vi "Database Viewer.vi"() -> ()   [LabVIEW 2019, in "Database Viewer.lvclass"]
doc: "- key stroke \"Left\" = \"Ctrl\" + \"Left\", \"Right\" = \"Ctrl\" + \"Right\" since left and right arror key are often used and using them for event will intertere with cursor movement.\n- drag cursor will update the start and end\n- load favorite A by Ctrl + A (?)\n- load favorite B by Ctrl + B (?)\n- load favorite C by Ctrl + C (?)"
uses:
  Database Viewer.lvclass
  typedefs/Time Mode--enum.ctl
  typedefs/Time Bucket--enum.ctl
  <vilib>/Utility/miscctls.llb/LVRangeTypeDef.ctl
  <userlib>/LevyLab/Instrument Framework/SMOs/Configuration/Configuration.lvclass
  typedefs/UI Controls--cluster.ctl
  Database Viewer.lvclass/Database Viewer.ctl
  <vilib>/Utility/miscctls.llb/LVRectTypeDef.ctl
  <vilib>/Utility/sysdir.llb/System Directory Type.ctl
  <userlib>/_OpenG.lib/array/array.llb/Index 1D Array Elements (String)__ogtk.vi
  <userlib>/LevyLab/LV-Data/LV-Data.PG/LV-Data.PGSQL.lvclass
  <userlib>/LevyLab/LV-Data/LV-Data.ITX/LV-Data.ITX.lvclass
  <userlib>/LevyLab/Instrument Framework/SMOs/Instrument/Instrument.lvclass
panel:
  in  "Disconnect":bool
  in  "Exit":bool
  out "Status":string
  in  "Time Bucket":T1=enum."automatic"
  out "Get Trace SQL":string
  in  "Execute Custom SQL?":bool
  in  "SQL String":string
  in  "Y Scale Mapping (Right)":enum16{"linear", "log"}(ring)
  in  "Max Points":i32=1000
  in  "Y Scale Mapping (Left)":enum16{"linear", "log"}(ring)
  in  "Median Filter?":bool
  in  "Favorite":enum16{"A", "B", "C"}(ring)
  in  "DST":bool=TRUE caption="Blank Button"
  in  "Variables (left axis)":u16[](array[ring]) caption="Display the following network shared variables (Left / Y)" items=["ALEX_DEMO: DEMO (discoveries)", "AML Gauges (Analysis): Emission Current (A)", "AML Gauges (Analysis): Fault ()", "AML Gauges (Analysis): IG Pressure (mbar)", "AML Gauges (Analysis): Instrument Status ()", "AML Gauges (Analysis): Pirani 1 Pressure (mbar)", "AML Gauges (Analysis): Pirani 2 Pressure (mbar)", "AML Gauges (Analysis): Relay A ()", "AML Gauges (Analysis): Relay B ()", "AML Gauges (Analysis): Relay C ()", "AML Gauges (Analysis): Relay D ()", "AML Gauges (Analysis): Trip A Association ()", "AML Gauges (Analysis): Trip A Pressure (mbar)", "AML Gauges (Analysis): Trip B Association ()", "AML Gauges (Analysis): Trip B Pressure (mbar)", "AML Gauges (Analysis): Trip C Association ()", "AML Gauges (Analysis): Trip C Pressure (mbar)", "AML Gauges (Analysis): Trip D Association ()", "AML Gauges (Analysis): Trip D Pressure (mbar)", "AML Gauges (Prep): Emission Current (A)", "AML Gauges (Prep): Fault ()", "AML Gauges (Prep): IG Pressure (mbar)", "AML Gauges (Prep): Instrument Status ()", "AML Gauges (Prep): Pirani 1 Pressure (mbar)", "AML Gauges (Prep): Pirani 2 Pressure (mbar)", "AML Gauges (Prep): Relay A ()", "AML Gauges (Prep): Relay B ()", "AML Gauges (Prep): Relay C ()", "AML Gauges (Prep): Relay D ()", "AML Gauges (Prep): Trip A Association ()", "AML Gauges (Prep): Trip A Pressure (mbar)", "AML Gauges (Prep): Trip B Association ()", "AML Gauges (Prep): Trip B Pressure (mbar)", "AML Gauges (Prep): Trip C Association ()", "AML Gauges (Prep): Trip C Pressure (mbar)", "AML Gauges (Prep): Trip D Association ()", "AML Gauges (Prep): Trip D Pressure (mbar)", "ASEQSpectra: Spectra ()", "Agilent AFM: Device ()", "Agilent AFM: Tip Voltage (volts)", "Agilent AFM: User ()", "Agilent AFM: X Pos (a.u.)", "Agilent AFM: Y Pos (a.u.)", "Agilent AFM: Z Pos (a.u.)", "CL SMS 18: Field (T)", "CL SMS 18: He Level (mm)", "CL SMS 18: Rate ()", "CL SMS 18: Target (T)", "CL SMS 18: Voltage (V)", "Colby: Delay (ps)", "Cypher: Comments ()", "Cypher: Device ()", "Cypher: Status ()", "Cypher: User ()", "DR200: 100 mK Plate R (Ohm)", "DR200: 100 mK Plate T (K)", "DR200: 4K Head R X55749 (Ohm)", "DR200: 4K Head R X55750 (Ohm)", "DR200: 4K Head T X55749 (K)", "DR200: 4K Head T X55750 (K)", "DR200: 70K Head R PT100 1 (Ohm)", "DR200: 70K Head R PT100 2 (Ohm)", "DR200: 70K Head T PT100 1 (K)", "DR200: 70K Head T PT100 2 (K)", "DR200: Dewar Pressure (mbar)", "DR200: Forepump Pressure (mbar)", "DR200: MC Heater (W)", "DR200: MC R RuO2 (Ohm)", "DR200: MC R X55751 (Ohm)", "DR200: MC T RuO2 (K)", "DR200: MC T X55751 (K)", "DR200: Mag Bottom R X48230 (Ohm)", "DR200: Mag Bottom R X52698 (Ohm)", "DR200: Mag Bottom T X48230 (K)", "DR200: Mag Bottom T X52698 (K)", "DR200: Mag Top R X48230 (Ohm)", "DR200: Mag Top R X52698 (Ohm)", "DR200: Mag Top T X48230 (K)", "DR200: Mag Top T X52698 (K)", "DR200: Magnet Field (T)", "DR200: Magnet Field Target (T)", "DR200: Magnet PS Current (A)", "DR200: Magnet PS Field (T)", "DR200: Magnet PS Voltage (V)", "DR200: Magnet Status Activity ()", "DR200: Magnet Status Mode ()", "DR200: Magnet Status Switch Heater ()", "DR200: Magnet Status System ()", "DR200: Magnet Target Rate (-)", "DR200: PT Current (A)", "DR200: PT Helium T (C)", "DR200: PT Oil T (C)", "DR200: PT Water In T (C)", "DR200: PT Water Out T (C)", "DR200: PressureFPSafety (Bar)", "DR200: PressureM1Condense (Bar)", "DR200: PressureM3Tank (Bar)", "DR200: Still Heater (W)", "DR200: Still Pressure (mBar)", "DR200: Still R (Ohm)", "DR200: Still T (K)", "Element 2: Diode Current Actual (A)", "Element 2: Diode Current Set (A)", "Element 2: Laser Status ()", "Element 2: Pump Power (W)", "Element 2: Startup/Shutdown Status ()", "Element 2: Temp: Control Unit (C)", "Element 2: Temp: Laser Head Pos1 (C)", "Element 2: Temp: Laser Head Pos2 (C)", "Element 2: Temp: Pump Chassis (C)", "Element 2: Temp: Pump Diodes (C)", "Element 2: Temp: Pump PCB (C)", "Element 2: Temp: Pump Tower (C)", "Gemini2: Device ()", "Gemini2: User ()", "JEOL: Device ()", "JEOL: User ()", "Leiden CF FP: Flow ()", "Leiden CF FP: MaxiGauge1 (mbar)", "Leiden CF FP: MaxiGauge2 (mbar)", "Leiden CF FP: MaxiGauge3 (mbar)", "Leiden CF FP: MaxiGauge4 (mbar)", "Leiden CF FP: MaxiGauge5 (mbar)", "Leiden CF FP: MaxiGauge6 (mbar)", "Leiden CF FP: P1 (mbar)", "Leiden CF FP: P2 (mbar)", "Leiden CF FP: P3 (mbar)", "Leiden CF FP: P4 (mbar)", "Leiden CF FP: P5 (mbar)", "Leiden CF FP: P6 (mbar)", "Leiden CF FP: P7 (mbar)", "Leiden CF FP: PT Current (A)", "Leiden CF FP: PT Helium T (C)", "Leiden CF FP: PT Oil T (C)", "Leiden CF FP: PT On ()", "Leiden CF FP: PT P High (bar)", "Leiden CF FP: PT P Low (bar)", "Leiden CF FP: PT Water In T (C)", "Leiden CF FP: PT Water Out T (C)", "Leiden CF FP: STATE ()", "Leiden CF FP: state0 ()", "Leiden CF FP: state1 ()", "Leiden CF FP: state2 ()", "Leiden CF900: CF FP P1 (no_idea)", "Leiden CF900: CF_TC_I0 (Amp)", "Leiden CF900: CF_TC_I1 (Amp)", "Leiden CF900: CF_TC_I2 (Amp)", "Leiden CF900: CF_TC_I3 (Amp)", "Leiden CF900: CF_TC_R0 (ohms)", "Leiden CF900: CF_TC_R1 (ohms)", "Leiden CF900: CF_TC_R2 (ohms)", "Leiden CF900: CF_TC_R3 (ohms)", "Leiden CF900: CF_TC_R4 (ohms)", "Leiden CF900: CF_TC_R5 (ohms)", "Leiden CF900: CF_TC_R6 (ohms)", "Leiden CF900: CF_TC_R7 (ohms)", "Leiden CF900: CF_TC_T0 (mK)", "Leiden CF900: CF_TC_T1 (mK)", "Leiden CF900: CF_TC_T2 (mK)", "Leiden CF900: CF_TC_T3 (mK)", "Leiden CF900: CF_TC_T4 (mK)", "Leiden CF900: CF_TC_T5 (mK)", "Leiden CF900: CF_TC_T6 (mK)", "Leiden CF900: CF_TC_T7 (mK)", "Leiden CF900: CF_TC_Z_R0 (ohms)", "Leiden CF900: CF_TC_Z_R1 (ohms)", "Leiden CF900: CF_TC_Z_R2 (ohms)", "Leiden CF900: CF_TC_Z_R3 (ohms)", "Leiden CF900: CF_TC_Z_R4 (ohms)", "Leiden CF900: CF_TC_Z_R5 (ohms)", "Leiden CF900: CF_TC_Z_R6 (ohms)", "Leiden CF900: CF_TC_Z_R7 (ohms)", "Leiden CF900: CF_TC_Z_R8 (ohms)", "Leiden CF900: CF_TC_Z_R9 (ohms)", "Leiden CF900: CF_TC_Z_T0 (mK)", "Leiden CF900: CF_TC_Z_T1 (mK)", "Leiden CF900: CF_TC_Z_T2 (mK)", "Leiden CF900: CF_TC_Z_T3 (mK)", "Leiden CF900: CF_TC_Z_T4 (mK)", "Leiden CF900: CF_TC_Z_T5 (mK)", "Leiden CF900: CF_TC_Z_T6 (mK)", "Leiden CF900: CF_TC_Z_T7 (mK)", "Leiden CF900: CF_TC_Z_T8 (mK)", "Leiden CF900: CF_TC_Z_T9 (mK)", "Leiden CF900: CF_TC_Z_calibration ()", "Leiden CF900: CF_TC_Z_description ()", "Leiden CF900: CF_TC_calibration ()", "Leiden CF900: CF_TC_description ()", "Leiden CF900: Device ()", "Leiden CF900: User ()", "Leiden MNK Front Panel: Flow ()", "Leiden MNK Front Panel: MaxiGauge1 (mbar)", "Leiden MNK Front Panel: MaxiGauge2 (mbar)", "Leiden MNK Front Panel: MaxiGauge3 (mbar)", "Leiden MNK Front Panel: MaxiGauge4 (mbar)", "Leiden MNK Front Panel: MaxiGauge5 (mbar)", "Leiden MNK Front Panel: MaxiGauge6 (mbar)", "Leiden MNK Front Panel: P1 (mbar)", "Leiden MNK Front Panel: P2 (mbar)", "Leiden MNK Front Panel: P3 (mbar)", "Leiden MNK Front Panel: P4 (mbar)", "Leiden MNK Front Panel: P5 (mbar)", "Leiden MNK Front Panel: P6 (mbar)", "Leiden MNK Front Panel: P7 (mbar)", "Leiden MNK Front Panel: STATE ()", "Leiden MNK Front Panel: state0 ()", "Leiden MNK Front Panel: state1 ()", "Leiden MNK Front Panel: state2 ()", "MFP3D: Device ()", "MFP3D: User ()", "MNK_18T: Device ()", "MNK_18T: IPS Command ()", "MNK_18T: IPS Current (A)", "MNK_18T: IPS IPS Voltage (V)", "MNK_18T: IPS LHe (%)", "MNK_18T: IPS LN2 (%)", "MNK_18T: IPS M1 Current (A)", "MNK_18T: IPS M1 Voltage (V)", "MNK_18T: IPS M2 Current (A)", "MNK_18T: IPS M2 Voltage (V)", "MNK_18T: IPS M3 Current (A)", "MNK_18T: IPS M3 Voltage (V)", "MNK_18T: IPS Magnet Field (T)", "MNK_18T: IPS PS Field (T)", "MNK_18T: IPS Reply ()", "MNK_18T: IPS Status ()", "MNK_18T: IPS Switch ()", "MNK_18T: IPS Target Field (T)", "MNK_18T: IPS Target Field Rate (T/min)", "MNK_18T: IPS Temperature (K)", "MNK_18T: IPS Temperature Resistance (Ohms)", "MNK_18T: ITC Command ()", "MNK_18T: ITC Needle Valve (%)", "MNK_18T: ITC Pressure (mbar)", "MNK_18T: ITC Reply ()", "MNK_18T: ITC Temperature (K)", "MNK_18T: ITC Temperature R (Ohms)", "MNK_18T: MNK_CMN-187_T (mK)", "MNK_18T: MNK_CMN-187_Z (H)", "MNK_18T: MNK_Cstill_T (mK)", "MNK_18T: MNK_Cstill_Z (pF)", "MNK_18T: MNK_TC_I0 (Amp)", "MNK_18T: MNK_TC_I1 (Amp)", "MNK_18T: MNK_TC_I2 (Amp)", "MNK_18T: MNK_TC_I3 (Amp)", "MNK_18T: MNK_TC_R0 (ohms)", "MNK_18T: MNK_TC_R1 (ohms)", "MNK_18T: MNK_TC_R2 (ohms)", "MNK_18T: MNK_TC_R3 (ohms)", "MNK_18T: MNK_TC_R4 (ohms)", "MNK_18T: MNK_TC_R5 (ohms)", "MNK_18T: MNK_TC_R6 (ohms)", "MNK_18T: MNK_TC_R7 (ohms)", "MNK_18T: MNK_TC_T0 (mK)", "MNK_18T: MNK_TC_T1 (mK)", "MNK_18T: MNK_TC_T2 (mK)", "MNK_18T: MNK_TC_T3 (mK)", "MNK_18T: MNK_TC_T4 (mK)", "MNK_18T: MNK_TC_T5 (mK)", "MNK_18T: MNK_TC_T6 (mK)", "MNK_18T: MNK_TC_T7 (mK)", "MNK_18T: MNK_TC_calibration ()", "MNK_18T: MNK_TC_description ()", "MNK_18T: User ()", "Montana Cryostation: Alarm State ()", "Montana Cryostation: Case Valve State ()", "Montana Cryostation: Chamber Pressure (mTorr)", "Montana Cryostation: Cold Head Speed (Hz)", "Montana Cryostation: Compressor Return Pressure (MPa)", "Montana Cryostation: Compressor Run State ()", "Montana Cryostation: Compressor Speed (Hz)", "Montana Cryostation: Compressor Supply Pressure (MPa)", "Montana Cryostation: Device ()", "Montana Cryostation: Idle State ()", "Montana Cryostation: Nitrogen State ()", "Montana Cryostation: Platform Heater Power (W)", "Montana Cryostation: Platform Stability (K)", "Montana Cryostation: Platform Temperature (K)", "Montana Cryostation: Sample Stability (K)", "Montana Cryostation: Sample Temperature (K)", "Montana Cryostation: Stage 1 Heater Power (W)", "Montana Cryostation: Stage 1 Temperature (K)", "Montana Cryostation: Stage 2 Heater Power (W)", "Montana Cryostation: Stage 2 Temperature (K)", "Montana Cryostation: Temperature Set Point (K)", "Montana Cryostation: User ()", "Montana Cryostation: User Stability (K)", "Montana Cryostation: User Temperature (K)", "Montana Cryostation: User Temperature Set Point (K)", "Montana Cryostation: Vent Valve State ()", "Oxford VRM: Current PSU 1 (A)", "Oxford VRM: Current PSU 2 (A)", "Oxford VRM: Current PSU 3 (A)", "Oxford VRM: Current PSU 4 (A)", "Oxford VRM: Current PSU 5 (A)", "Oxford VRM: Current PSU 6 (A)", "Oxford VRM: Current X (A)", "Oxford VRM: Current Y (A)", "Oxford VRM: Current Z (A)", "Oxford VRM: Field X (T)", "Oxford VRM: Field Y (T)", "Oxford VRM: Field Z (T)", "Oxford VRM: IPS Reply ()", "Oxford VRM: Status X ()", "Oxford VRM: Status Y ()", "Oxford VRM: Status Z ()", "Oxford VRM: Target Field Rate X (T/min)", "Oxford VRM: Target Field Rate Y (T/min)", "Oxford VRM: Target Field Rate Z (T/min)", "Oxford VRM: Target Field X (T)", "Oxford VRM: Target Field Y (T)", "Oxford VRM: Target Field Z (T)", "Oxford VRM: Voltage PSU 1 (V)", "Oxford VRM: Voltage PSU 2 (V)", "Oxford VRM: Voltage PSU 3 (V)", "Oxford VRM: Voltage PSU 4 (V)", "Oxford VRM: Voltage PSU 5 (V)", "Oxford VRM: Voltage PSU 6 (V)", "Oxford VRM: Voltage X (V)", "Oxford VRM: Voltage Y (V)", "Oxford VRM: Voltage Z (V)", "PPMS 1: Chamber Status ()", "PPMS 1: Device ()", "PPMS 1: Helium Level (%)", "PPMS 1: Magnet Status ()", "PPMS 1: Magnetic Field (Oe)", "PPMS 1: Position (deg)", "PPMS 1: Temperature (K)", "PPMS 1: Temperature Status ()", "PPMS 1: User ()", "PPMS 2: Chamber Status ()", "PPMS 2: Device ()", "PPMS 2: Helium Level (%)", "PPMS 2: Magnet Status ()", "PPMS 2: Magnetic Field (Oe)", "PPMS 2: Position (deg)", "PPMS 2: Temperature (K)", "PPMS 2: Temperature Status ()", "PPMS 2: User ()", "PPMS 3: Chamber Status ()", "PPMS 3: Device ()", "PPMS 3: Helium Level (%)", "PPMS 3: Magnet Status ()", "PPMS 3: Magnetic Field (T)", "PPMS 3: Temperature (K)", "PPMS 3: Temperature Status ()", "PPMS 3: User ()", "PPMSim: Chamber Status ()", "PPMSim: Device ()", "PPMSim: Helium Level (%)", "PPMSim: Loaded? ()", "PPMSim: Magnet Status ()", "PPMSim: Magnetic Field (T)", "PPMSim: No. of leads (leads)", "PPMSim: Temperature (K)", "PPMSim: Temperature Status ()", "PPMSim: User ()", "PPMSim: v1 (volts)", "PPMSim: v2 (volts)", "PPMSim: v3 (volts)", "Pfeiffer ASM340: Leak Rate (mbar.l/s)", "Pfeiffer ASM340: Pressure (mbar)", "Razorbill: Bridge Capacitance (pF)", "Razorbill: Bridge Excitation (V)", "Razorbill: Bridge Loss (nS)", "Razorbill: Current Ch 1 (A)", "Razorbill: Current Ch 2 (A)", "Razorbill: Level Ch 1 (V)", "Razorbill: Level Ch 2 (V)", "Razorbill: Output State Ch 1 ()", "Razorbill: Output State Ch 2 ()", "Razorbill: Slew Ch 1 (V/s)", "Razorbill: Slew Ch 2 (V/s)", "Razorbill: Voltage Ch 1 (V)", "Razorbill: Voltage Ch 2 (V)", "T/H Monitoring:  (K)", "T/H Monitoring: Astartes_H (%RH)", "T/H Monitoring: Astartes_T (K)", "T/H Monitoring: Centaur_H (%RH)", "T/H Monitoring: Centaur_T (K)", "T/H Monitoring: CustardPie_H (%RH)", "T/H Monitoring: CustardPie_T (K)", "T/H Monitoring: DOT_H (%RH)", "T/H Monitoring: DOT_T (K)", "T/H Monitoring: Griffin_H (%RH)", "T/H Monitoring: Griffin_T (K)", "T/H Monitoring: Kholek_H (%RH)", "T/H Monitoring: Kholek_T (K)", "T/H Monitoring: MFP3D2_H (%RH)", "T/H Monitoring: MFP3D2_T (K)", "T/H Monitoring: MFP3D_H (%RH)", "T/H Monitoring: MFP3D_T (K)", "TEST_TABLE:  (K)", "TEST_TABLE: Columntest2 ()", "TEST_TABLE: Columntest3 ()", "TEST_TABLE: Columntest4 ()", "TEST_TABLE: Custard_T (K)", "TEST_TABLE: Kholek_T (K)", "TEST_TABLE: MFP3D2.phyast.pitt.edu_H (%RH)", "TEST_TABLE: MFP3D2.phyast.pitt.edu_T (K)", "TEST_TABLE: MFP3D2_H (%RH)", "TEST_TABLE: MFP3D2_T (K)", "TEST_TABLE: ON? ()", "TEST_TABLE: Ranjani_H (%)", "TEST_TABLE: Ranjani_T (K)", "TEST_TABLE: Ranjani_new (K)", "TEST_TABLE: Temperature (Kelvin)", "TEST_TABLE: Temperhum_H (%RH)", "TEST_TABLE: Temperhum_T (K)", "TEST_TABLE: Test (tests)", "TEST_TABLE: Test2 (tests)", "TEST_TABLE: _H (%RH)", "TEST_TABLE: _T (K)", "TEST_TABLE: col5 ()", "TEST_TABLE: column2 ()", "TEST_TABLE: connected ()", "TEST_TABLE: ranjani_1 (discoveries)", "TEST_TABLE: sample ()", "TEST_TABLE: test (K)", "TEST_TABLE: testcolumn3 ()", "TEST_TABLE: user ()", "TEST_TABLE: voltaga__demo (volts)", "TEST_TABLE: voltage 2 (volts)", "TEST_TABLE_2: Columntest7 ()", "TEST_TABLE_2: columntest4 ()", "TEST_TABLE_2: new column name (elias)", "TEST_TABLE_2: successfulness (discoveries)", "THz1 SPC: DummyData ()", "Tsunami: Device ()", "Tsunami: User ()"]
  in  "Variables (right axis)":u16[](array[ring]) caption="Display the following network shared variables (Right / X)" items=["ALEX_DEMO: DEMO (discoveries)", "AML Gauges (Analysis): Emission Current (A)", "AML Gauges (Analysis): Fault ()", "AML Gauges (Analysis): IG Pressure (mbar)", "AML Gauges (Analysis): Instrument Status ()", "AML Gauges (Analysis): Pirani 1 Pressure (mbar)", "AML Gauges (Analysis): Pirani 2 Pressure (mbar)", "AML Gauges (Analysis): Relay A ()", "AML Gauges (Analysis): Relay B ()", "AML Gauges (Analysis): Relay C ()", "AML Gauges (Analysis): Relay D ()", "AML Gauges (Analysis): Trip A Association ()", "AML Gauges (Analysis): Trip A Pressure (mbar)", "AML Gauges (Analysis): Trip B Association ()", "AML Gauges (Analysis): Trip B Pressure (mbar)", "AML Gauges (Analysis): Trip C Association ()", "AML Gauges (Analysis): Trip C Pressure (mbar)", "AML Gauges (Analysis): Trip D Association ()", "AML Gauges (Analysis): Trip D Pressure (mbar)", "AML Gauges (Prep): Emission Current (A)", "AML Gauges (Prep): Fault ()", "AML Gauges (Prep): IG Pressure (mbar)", "AML Gauges (Prep): Instrument Status ()", "AML Gauges (Prep): Pirani 1 Pressure (mbar)", "AML Gauges (Prep): Pirani 2 Pressure (mbar)", "AML Gauges (Prep): Relay A ()", "AML Gauges (Prep): Relay B ()", "AML Gauges (Prep): Relay C ()", "AML Gauges (Prep): Relay D ()", "AML Gauges (Prep): Trip A Association ()", "AML Gauges (Prep): Trip A Pressure (mbar)", "AML Gauges (Prep): Trip B Association ()", "AML Gauges (Prep): Trip B Pressure (mbar)", "AML Gauges (Prep): Trip C Association ()", "AML Gauges (Prep): Trip C Pressure (mbar)", "AML Gauges (Prep): Trip D Association ()", "AML Gauges (Prep): Trip D Pressure (mbar)", "ASEQSpectra: Spectra ()", "Agilent AFM: Device ()", "Agilent AFM: Tip Voltage (volts)", "Agilent AFM: User ()", "Agilent AFM: X Pos (a.u.)", "Agilent AFM: Y Pos (a.u.)", "Agilent AFM: Z Pos (a.u.)", "CL SMS 18: Field (T)", "CL SMS 18: He Level (mm)", "CL SMS 18: Rate ()", "CL SMS 18: Target (T)", "CL SMS 18: Voltage (V)", "Colby: Delay (ps)", "Cypher: Comments ()", "Cypher: Device ()", "Cypher: Status ()", "Cypher: User ()", "DR200: 100 mK Plate R (Ohm)", "DR200: 100 mK Plate T (K)", "DR200: 4K Head R X55749 (Ohm)", "DR200: 4K Head R X55750 (Ohm)", "DR200: 4K Head T X55749 (K)", "DR200: 4K Head T X55750 (K)", "DR200: 70K Head R PT100 1 (Ohm)", "DR200: 70K Head R PT100 2 (Ohm)", "DR200: 70K Head T PT100 1 (K)", "DR200: 70K Head T PT100 2 (K)", "DR200: Dewar Pressure (mbar)", "DR200: Forepump Pressure (mbar)", "DR200: MC Heater (W)", "DR200: MC R RuO2 (Ohm)", "DR200: MC R X55751 (Ohm)", "DR200: MC T RuO2 (K)", "DR200: MC T X55751 (K)", "DR200: Mag Bottom R X48230 (Ohm)", "DR200: Mag Bottom R X52698 (Ohm)", "DR200: Mag Bottom T X48230 (K)", "DR200: Mag Bottom T X52698 (K)", "DR200: Mag Top R X48230 (Ohm)", "DR200: Mag Top R X52698 (Ohm)", "DR200: Mag Top T X48230 (K)", "DR200: Mag Top T X52698 (K)", "DR200: Magnet Field (T)", "DR200: Magnet Field Target (T)", "DR200: Magnet PS Current (A)", "DR200: Magnet PS Field (T)", "DR200: Magnet PS Voltage (V)", "DR200: Magnet Status Activity ()", "DR200: Magnet Status Mode ()", "DR200: Magnet Status Switch Heater ()", "DR200: Magnet Status System ()", "DR200: Magnet Target Rate (-)", "DR200: PT Current (A)", "DR200: PT Helium T (C)", "DR200: PT Oil T (C)", "DR200: PT Water In T (C)", "DR200: PT Water Out T (C)", "DR200: PressureFPSafety (Bar)", "DR200: PressureM1Condense (Bar)", "DR200: PressureM3Tank (Bar)", "DR200: Still Heater (W)", "DR200: Still Pressure (mBar)", "DR200: Still R (Ohm)", "DR200: Still T (K)", "Element 2: Diode Current Actual (A)", "Element 2: Diode Current Set (A)", "Element 2: Laser Status ()", "Element 2: Pump Power (W)", "Element 2: Startup/Shutdown Status ()", "Element 2: Temp: Control Unit (C)", "Element 2: Temp: Laser Head Pos1 (C)", "Element 2: Temp: Laser Head Pos2 (C)", "Element 2: Temp: Pump Chassis (C)", "Element 2: Temp: Pump Diodes (C)", "Element 2: Temp: Pump PCB (C)", "Element 2: Temp: Pump Tower (C)", "Gemini2: Device ()", "Gemini2: User ()", "JEOL: Device ()", "JEOL: User ()", "Leiden CF FP: Flow ()", "Leiden CF FP: MaxiGauge1 (mbar)", "Leiden CF FP: MaxiGauge2 (mbar)", "Leiden CF FP: MaxiGauge3 (mbar)", "Leiden CF FP: MaxiGauge4 (mbar)", "Leiden CF FP: MaxiGauge5 (mbar)", "Leiden CF FP: MaxiGauge6 (mbar)", "Leiden CF FP: P1 (mbar)", "Leiden CF FP: P2 (mbar)", "Leiden CF FP: P3 (mbar)", "Leiden CF FP: P4 (mbar)", "Leiden CF FP: P5 (mbar)", "Leiden CF FP: P6 (mbar)", "Leiden CF FP: P7 (mbar)", "Leiden CF FP: PT Current (A)", "Leiden CF FP: PT Helium T (C)", "Leiden CF FP: PT Oil T (C)", "Leiden CF FP: PT On ()", "Leiden CF FP: PT P High (bar)", "Leiden CF FP: PT P Low (bar)", "Leiden CF FP: PT Water In T (C)", "Leiden CF FP: PT Water Out T (C)", "Leiden CF FP: STATE ()", "Leiden CF FP: state0 ()", "Leiden CF FP: state1 ()", "Leiden CF FP: state2 ()", "Leiden CF900: CF FP P1 (no_idea)", "Leiden CF900: CF_TC_I0 (Amp)", "Leiden CF900: CF_TC_I1 (Amp)", "Leiden CF900: CF_TC_I2 (Amp)", "Leiden CF900: CF_TC_I3 (Amp)", "Leiden CF900: CF_TC_R0 (ohms)", "Leiden CF900: CF_TC_R1 (ohms)", "Leiden CF900: CF_TC_R2 (ohms)", "Leiden CF900: CF_TC_R3 (ohms)", "Leiden CF900: CF_TC_R4 (ohms)", "Leiden CF900: CF_TC_R5 (ohms)", "Leiden CF900: CF_TC_R6 (ohms)", "Leiden CF900: CF_TC_R7 (ohms)", "Leiden CF900: CF_TC_T0 (mK)", "Leiden CF900: CF_TC_T1 (mK)", "Leiden CF900: CF_TC_T2 (mK)", "Leiden CF900: CF_TC_T3 (mK)", "Leiden CF900: CF_TC_T4 (mK)", "Leiden CF900: CF_TC_T5 (mK)", "Leiden CF900: CF_TC_T6 (mK)", "Leiden CF900: CF_TC_T7 (mK)", "Leiden CF900: CF_TC_Z_R0 (ohms)", "Leiden CF900: CF_TC_Z_R1 (ohms)", "Leiden CF900: CF_TC_Z_R2 (ohms)", "Leiden CF900: CF_TC_Z_R3 (ohms)", "Leiden CF900: CF_TC_Z_R4 (ohms)", "Leiden CF900: CF_TC_Z_R5 (ohms)", "Leiden CF900: CF_TC_Z_R6 (ohms)", "Leiden CF900: CF_TC_Z_R7 (ohms)", "Leiden CF900: CF_TC_Z_R8 (ohms)", "Leiden CF900: CF_TC_Z_R9 (ohms)", "Leiden CF900: CF_TC_Z_T0 (mK)", "Leiden CF900: CF_TC_Z_T1 (mK)", "Leiden CF900: CF_TC_Z_T2 (mK)", "Leiden CF900: CF_TC_Z_T3 (mK)", "Leiden CF900: CF_TC_Z_T4 (mK)", "Leiden CF900: CF_TC_Z_T5 (mK)", "Leiden CF900: CF_TC_Z_T6 (mK)", "Leiden CF900: CF_TC_Z_T7 (mK)", "Leiden CF900: CF_TC_Z_T8 (mK)", "Leiden CF900: CF_TC_Z_T9 (mK)", "Leiden CF900: CF_TC_Z_calibration ()", "Leiden CF900: CF_TC_Z_description ()", "Leiden CF900: CF_TC_calibration ()", "Leiden CF900: CF_TC_description ()", "Leiden CF900: Device ()", "Leiden CF900: User ()", "Leiden MNK Front Panel: Flow ()", "Leiden MNK Front Panel: MaxiGauge1 (mbar)", "Leiden MNK Front Panel: MaxiGauge2 (mbar)", "Leiden MNK Front Panel: MaxiGauge3 (mbar)", "Leiden MNK Front Panel: MaxiGauge4 (mbar)", "Leiden MNK Front Panel: MaxiGauge5 (mbar)", "Leiden MNK Front Panel: MaxiGauge6 (mbar)", "Leiden MNK Front Panel: P1 (mbar)", "Leiden MNK Front Panel: P2 (mbar)", "Leiden MNK Front Panel: P3 (mbar)", "Leiden MNK Front Panel: P4 (mbar)", "Leiden MNK Front Panel: P5 (mbar)", "Leiden MNK Front Panel: P6 (mbar)", "Leiden MNK Front Panel: P7 (mbar)", "Leiden MNK Front Panel: STATE ()", "Leiden MNK Front Panel: state0 ()", "Leiden MNK Front Panel: state1 ()", "Leiden MNK Front Panel: state2 ()", "MFP3D: Device ()", "MFP3D: User ()", "MNK_18T: Device ()", "MNK_18T: IPS Command ()", "MNK_18T: IPS Current (A)", "MNK_18T: IPS IPS Voltage (V)", "MNK_18T: IPS LHe (%)", "MNK_18T: IPS LN2 (%)", "MNK_18T: IPS M1 Current (A)", "MNK_18T: IPS M1 Voltage (V)", "MNK_18T: IPS M2 Current (A)", "MNK_18T: IPS M2 Voltage (V)", "MNK_18T: IPS M3 Current (A)", "MNK_18T: IPS M3 Voltage (V)", "MNK_18T: IPS Magnet Field (T)", "MNK_18T: IPS PS Field (T)", "MNK_18T: IPS Reply ()", "MNK_18T: IPS Status ()", "MNK_18T: IPS Switch ()", "MNK_18T: IPS Target Field (T)", "MNK_18T: IPS Target Field Rate (T/min)", "MNK_18T: IPS Temperature (K)", "MNK_18T: IPS Temperature Resistance (Ohms)", "MNK_18T: ITC Command ()", "MNK_18T: ITC Needle Valve (%)", "MNK_18T: ITC Pressure (mbar)", "MNK_18T: ITC Reply ()", "MNK_18T: ITC Temperature (K)", "MNK_18T: ITC Temperature R (Ohms)", "MNK_18T: MNK_CMN-187_T (mK)", "MNK_18T: MNK_CMN-187_Z (H)", "MNK_18T: MNK_Cstill_T (mK)", "MNK_18T: MNK_Cstill_Z (pF)", "MNK_18T: MNK_TC_I0 (Amp)", "MNK_18T: MNK_TC_I1 (Amp)", "MNK_18T: MNK_TC_I2 (Amp)", "MNK_18T: MNK_TC_I3 (Amp)", "MNK_18T: MNK_TC_R0 (ohms)", "MNK_18T: MNK_TC_R1 (ohms)", "MNK_18T: MNK_TC_R2 (ohms)", "MNK_18T: MNK_TC_R3 (ohms)", "MNK_18T: MNK_TC_R4 (ohms)", "MNK_18T: MNK_TC_R5 (ohms)", "MNK_18T: MNK_TC_R6 (ohms)", "MNK_18T: MNK_TC_R7 (ohms)", "MNK_18T: MNK_TC_T0 (mK)", "MNK_18T: MNK_TC_T1 (mK)", "MNK_18T: MNK_TC_T2 (mK)", "MNK_18T: MNK_TC_T3 (mK)", "MNK_18T: MNK_TC_T4 (mK)", "MNK_18T: MNK_TC_T5 (mK)", "MNK_18T: MNK_TC_T6 (mK)", "MNK_18T: MNK_TC_T7 (mK)", "MNK_18T: MNK_TC_calibration ()", "MNK_18T: MNK_TC_description ()", "MNK_18T: User ()", "Montana Cryostation: Alarm State ()", "Montana Cryostation: Case Valve State ()", "Montana Cryostation: Chamber Pressure (mTorr)", "Montana Cryostation: Cold Head Speed (Hz)", "Montana Cryostation: Compressor Return Pressure (MPa)", "Montana Cryostation: Compressor Run State ()", "Montana Cryostation: Compressor Speed (Hz)", "Montana Cryostation: Compressor Supply Pressure (MPa)", "Montana Cryostation: Device ()", "Montana Cryostation: Idle State ()", "Montana Cryostation: Nitrogen State ()", "Montana Cryostation: Platform Heater Power (W)", "Montana Cryostation: Platform Stability (K)", "Montana Cryostation: Platform Temperature (K)", "Montana Cryostation: Sample Stability (K)", "Montana Cryostation: Sample Temperature (K)", "Montana Cryostation: Stage 1 Heater Power (W)", "Montana Cryostation: Stage 1 Temperature (K)", "Montana Cryostation: Stage 2 Heater Power (W)", "Montana Cryostation: Stage 2 Temperature (K)", "Montana Cryostation: Temperature Set Point (K)", "Montana Cryostation: User ()", "Montana Cryostation: User Stability (K)", "Montana Cryostation: User Temperature (K)", "Montana Cryostation: User Temperature Set Point (K)", "Montana Cryostation: Vent Valve State ()", "Oxford VRM: Current PSU 1 (A)", "Oxford VRM: Current PSU 2 (A)", "Oxford VRM: Current PSU 3 (A)", "Oxford VRM: Current PSU 4 (A)", "Oxford VRM: Current PSU 5 (A)", "Oxford VRM: Current PSU 6 (A)", "Oxford VRM: Current X (A)", "Oxford VRM: Current Y (A)", "Oxford VRM: Current Z (A)", "Oxford VRM: Field X (T)", "Oxford VRM: Field Y (T)", "Oxford VRM: Field Z (T)", "Oxford VRM: IPS Reply ()", "Oxford VRM: Status X ()", "Oxford VRM: Status Y ()", "Oxford VRM: Status Z ()", "Oxford VRM: Target Field Rate X (T/min)", "Oxford VRM: Target Field Rate Y (T/min)", "Oxford VRM: Target Field Rate Z (T/min)", "Oxford VRM: Target Field X (T)", "Oxford VRM: Target Field Y (T)", "Oxford VRM: Target Field Z (T)", "Oxford VRM: Voltage PSU 1 (V)", "Oxford VRM: Voltage PSU 2 (V)", "Oxford VRM: Voltage PSU 3 (V)", "Oxford VRM: Voltage PSU 4 (V)", "Oxford VRM: Voltage PSU 5 (V)", "Oxford VRM: Voltage PSU 6 (V)", "Oxford VRM: Voltage X (V)", "Oxford VRM: Voltage Y (V)", "Oxford VRM: Voltage Z (V)", "PPMS 1: Chamber Status ()", "PPMS 1: Device ()", "PPMS 1: Helium Level (%)", "PPMS 1: Magnet Status ()", "PPMS 1: Magnetic Field (Oe)", "PPMS 1: Position (deg)", "PPMS 1: Temperature (K)", "PPMS 1: Temperature Status ()", "PPMS 1: User ()", "PPMS 2: Chamber Status ()", "PPMS 2: Device ()", "PPMS 2: Helium Level (%)", "PPMS 2: Magnet Status ()", "PPMS 2: Magnetic Field (Oe)", "PPMS 2: Position (deg)", "PPMS 2: Temperature (K)", "PPMS 2: Temperature Status ()", "PPMS 2: User ()", "PPMS 3: Chamber Status ()", "PPMS 3: Device ()", "PPMS 3: Helium Level (%)", "PPMS 3: Magnet Status ()", "PPMS 3: Magnetic Field (T)", "PPMS 3: Temperature (K)", "PPMS 3: Temperature Status ()", "PPMS 3: User ()", "PPMSim: Chamber Status ()", "PPMSim: Device ()", "PPMSim: Helium Level (%)", "PPMSim: Loaded? ()", "PPMSim: Magnet Status ()", "PPMSim: Magnetic Field (T)", "PPMSim: No. of leads (leads)", "PPMSim: Temperature (K)", "PPMSim: Temperature Status ()", "PPMSim: User ()", "PPMSim: v1 (volts)", "PPMSim: v2 (volts)", "PPMSim: v3 (volts)", "Pfeiffer ASM340: Leak Rate (mbar.l/s)", "Pfeiffer ASM340: Pressure (mbar)", "Razorbill: Bridge Capacitance (pF)", "Razorbill: Bridge Excitation (V)", "Razorbill: Bridge Loss (nS)", "Razorbill: Current Ch 1 (A)", "Razorbill: Current Ch 2 (A)", "Razorbill: Level Ch 1 (V)", "Razorbill: Level Ch 2 (V)", "Razorbill: Output State Ch 1 ()", "Razorbill: Output State Ch 2 ()", "Razorbill: Slew Ch 1 (V/s)", "Razorbill: Slew Ch 2 (V/s)", "Razorbill: Voltage Ch 1 (V)", "Razorbill: Voltage Ch 2 (V)", "T/H Monitoring:  (K)", "T/H Monitoring: Astartes_H (%RH)", "T/H Monitoring: Astartes_T (K)", "T/H Monitoring: Centaur_H (%RH)", "T/H Monitoring: Centaur_T (K)", "T/H Monitoring: CustardPie_H (%RH)", "T/H Monitoring: CustardPie_T (K)", "T/H Monitoring: DOT_H (%RH)", "T/H Monitoring: DOT_T (K)", "T/H Monitoring: Griffin_H (%RH)", "T/H Monitoring: Griffin_T (K)", "T/H Monitoring: Kholek_H (%RH)", "T/H Monitoring: Kholek_T (K)", "T/H Monitoring: MFP3D2_H (%RH)", "T/H Monitoring: MFP3D2_T (K)", "T/H Monitoring: MFP3D_H (%RH)", "T/H Monitoring: MFP3D_T (K)", "TEST_TABLE:  (K)", "TEST_TABLE: Columntest2 ()", "TEST_TABLE: Columntest3 ()", "TEST_TABLE: Columntest4 ()", "TEST_TABLE: Custard_T (K)", "TEST_TABLE: Kholek_T (K)", "TEST_TABLE: MFP3D2.phyast.pitt.edu_H (%RH)", "TEST_TABLE: MFP3D2.phyast.pitt.edu_T (K)", "TEST_TABLE: MFP3D2_H (%RH)", "TEST_TABLE: MFP3D2_T (K)", "TEST_TABLE: ON? ()", "TEST_TABLE: Ranjani_H (%)", "TEST_TABLE: Ranjani_T (K)", "TEST_TABLE: Ranjani_new (K)", "TEST_TABLE: Temperature (Kelvin)", "TEST_TABLE: Temperhum_H (%RH)", "TEST_TABLE: Temperhum_T (K)", "TEST_TABLE: Test (tests)", "TEST_TABLE: Test2 (tests)", "TEST_TABLE: _H (%RH)", "TEST_TABLE: _T (K)", "TEST_TABLE: col5 ()", "TEST_TABLE: column2 ()", "TEST_TABLE: connected ()", "TEST_TABLE: ranjani_1 (discoveries)", "TEST_TABLE: sample ()", "TEST_TABLE: test (K)", "TEST_TABLE: testcolumn3 ()", "TEST_TABLE: user ()", "TEST_TABLE: voltaga__demo (volts)", "TEST_TABLE: voltage 2 (volts)", "TEST_TABLE_2: Columntest7 ()", "TEST_TABLE_2: columntest4 ()", "TEST_TABLE_2: new column name (elias)", "TEST_TABLE_2: successfulness (discoveries)", "THz1 SPC: DummyData ()", "Tsunami: Device ()", "Tsunami: User ()"]
  in  "Export Button":bool
  in  "export path":path=path "C:/Users/Voodoo/Desktop/export"
  out "Shift Hours":dbl=-4.0 format="%#_13g"
  in  "Igor":bool=TRUE caption="Blank Button"
  in  "Connect":bool
  in  "Save Configuration":bool
  in  "Load Configuration":bool
  in  "Mode":T2
  in  "Span":dbl format="%<%D d %H hr %M min %S s>t"
  in  "Trees Visible? >>>>>>":bool
  in  "Tab Control":T3(tab)
  out "Database Time Graph":T4(graph) caption="Retrieved from Citadel 5"
  out "XY Graph":cluster{"data":dbl[], "data":dbl[]}[](graph)
  out "SQL Result":string[][](table)
  out "Trigger Timer (ms)":u32
  out "\"\"":string="Exit\nData: Cleanup\nPostgres: Close Connection\nMacro: Exit\n\nUI: Hide/show trees\nData: Set timeout\nUI: Front Panel State\nUI: Initialize\nInitialize Core Data\nData: Initialize\nMacro: Initialize\r\n"
  in  "Start":dbl format="%<%x %.3X>T"
  in  "End":dbl format="%<%x %.3X>T"
  in  "Seek Back Button":bool
  in  "Seek Forward Button":bool
  in  "Seek":dbl=3600.0 format="%<%H:%M:%S>t"
  in  "Tab Control 2":enum32{"TimeScale - Tree"}(tab)
  in  "postgreSQL Tree (Right / X)":string[](tree)
  in  "postgreSQL Tree (Left / Y)":string[](tree)
  # "Database Connect"
  # "Traces"
  # "Configuration"
  # "Export"
  # "Information: LevyLab Database Viewer v2023.02.17"
  # "Time Axis"
  # "Vertical Axis"
  # "Custom SQL"
  # "Y1\nY2\n.\n.\n."
  # "X1\nX2\n.\n.\n."
  # "."
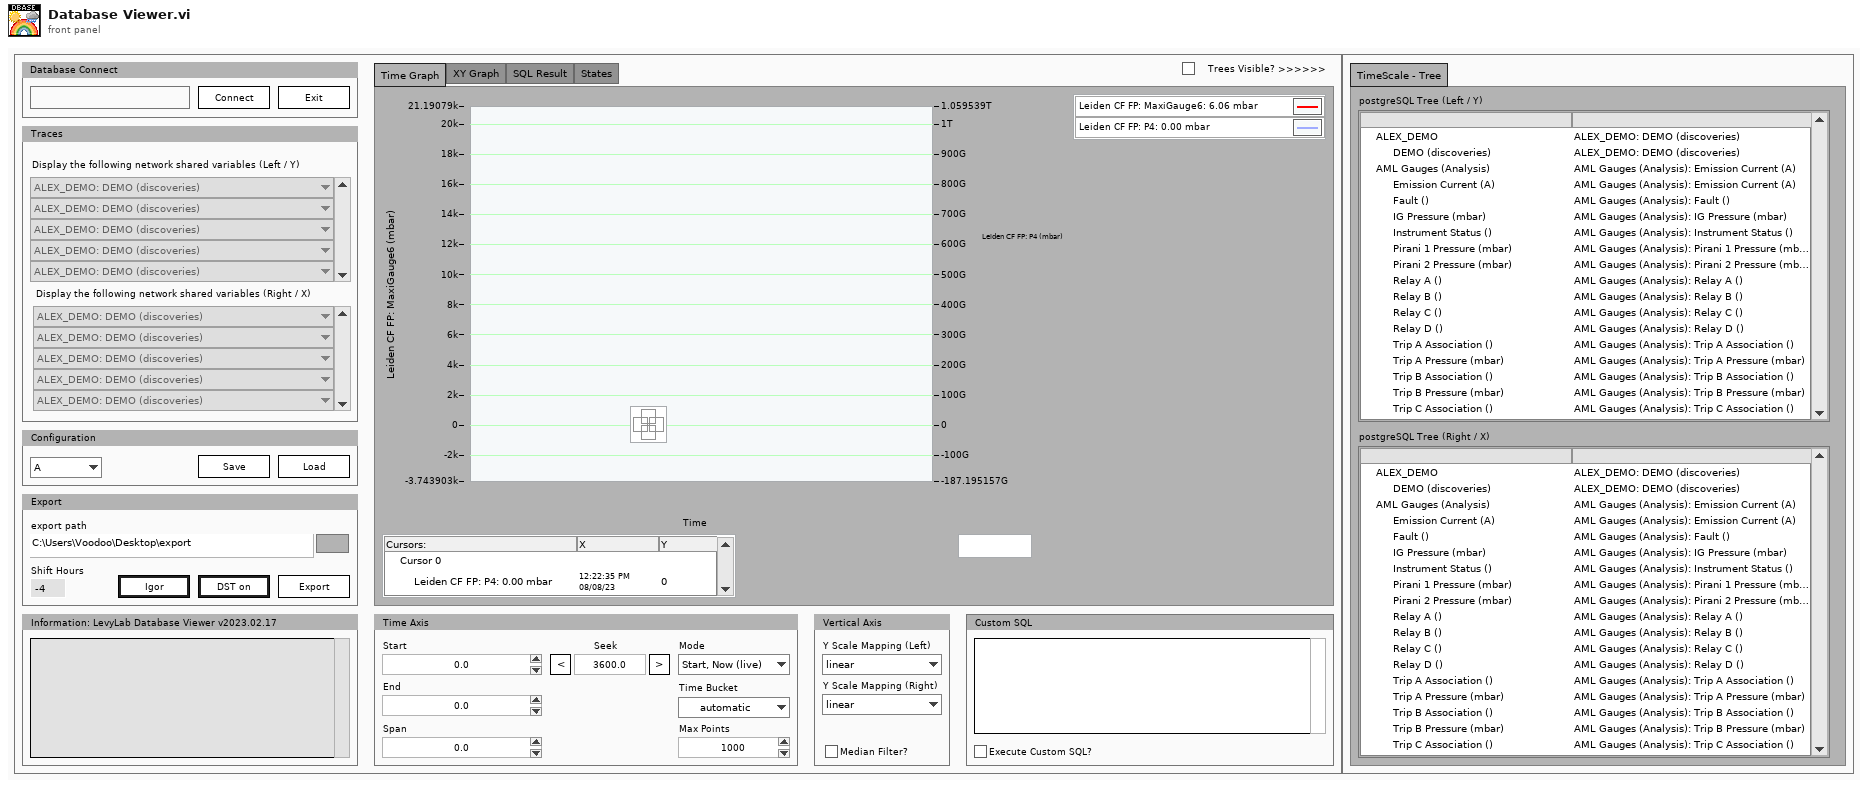
[diagram p1: front panel]
types:
  T1 = typedef "Database Viewer.lvclass/Time Bucket--enum.ctl" = enum16{"max points", "automatic", "1 second", "10 seconds", "1 minute", "10 minutes", "1 hour", "10 hours", "1 day", "10 days", "1 month"}
  T2 = typedef "Database Viewer.lvclass/Time Mode--enum.ctl" = enum16{"Start, Now (live)", "Start, End", "Start + Span", "End - Span"}
  T3 = enum32{"Time Graph", "XY Graph", "SQL Result", "States"}
  T4 = cluster{"timestamps":timestamp[], "data":dbl[]}[]
  T5 = enum32{"Invalid", "Standard", "Closed", "Hidden", "Minimized", "Maximized"}
  T6 = enum32{"invalid app kind", "Development System", "Run Time System", "Student Edition", "Embedded LabVIEW", "Evaluation", "Custom"}
  T7 = typedef "LVRectTypeDef.ctl" = cluster{"Left":i16, "Top":i16, "Right":i16, "Bottom":i16}
  T8 = typedef "Database Viewer.lvclass/UI Controls--cluster.ctl" = cluster{"Variables (left axis)":u16[], "Variables (right axis)":u16[], "Time Mode":T2, "Time Bucket":T1, "Start Time":timestamp, "End Time":timestamp, "Step Size":dbl, "Y Scale Mapping (left)":enum16{"linear", "log"}, "max points per trace (all)":i32, "Y Scale Mapping (right)":enum16{"linear", "log"}, "Filter?":bool, "export path":path, "DST":bool}
  T9 = typedef "LVRangeTypeDef.ctl" = cluster{"Minimum":dbl, "Maximum":dbl, "Increment":dbl, "Minor Increment":dbl, "Start":dbl}
  T10 = cluster{"Core":cluster{"Current VI Reference":refnum<vi>, "Close Panel on Exit?":bool}, "self reference":refnum<class "Database Viewer.lvclass">, "Configuration":refnum<class "Configuration.lvclass">, "Database":path, "Connect Time":timestamp, "Variable Names":string[], "Variable Paths":string[], "Traces":cluster{"timestamps":timestamp[], "data":dbl[]}[], "NewRange":T9, "Time Graph":refnum<vi>, "XY Graph":refnum<vi>, "Time Interval":cluster{"start timestamp":timestamp, "stop timestamp (now)":timestamp}, "Ring items":cluster{string, i32}[], "PG Variables":cluster{"Table Names":string[], "Table Paths":string[], "PG Columns":string[], "Columns (right)":string[], "PG Names":string[]}, "No. of non PG vars":i32, "Controls Cluster":T8, "Status":string}
  T11 = cluster{"Table Names":string[], "Table Paths":string[], "PG Columns":string[], "Columns (right)":string[], "PG Names":string[]}
  T12 = cluster{"start timestamp":timestamp, "stop timestamp (now)":timestamp}
  T13 = cluster{"Current VI Reference":refnum<vi>, "Close Panel on Exit?":bool}
  T14 = typedef "System Directory Type.ctl" = i32
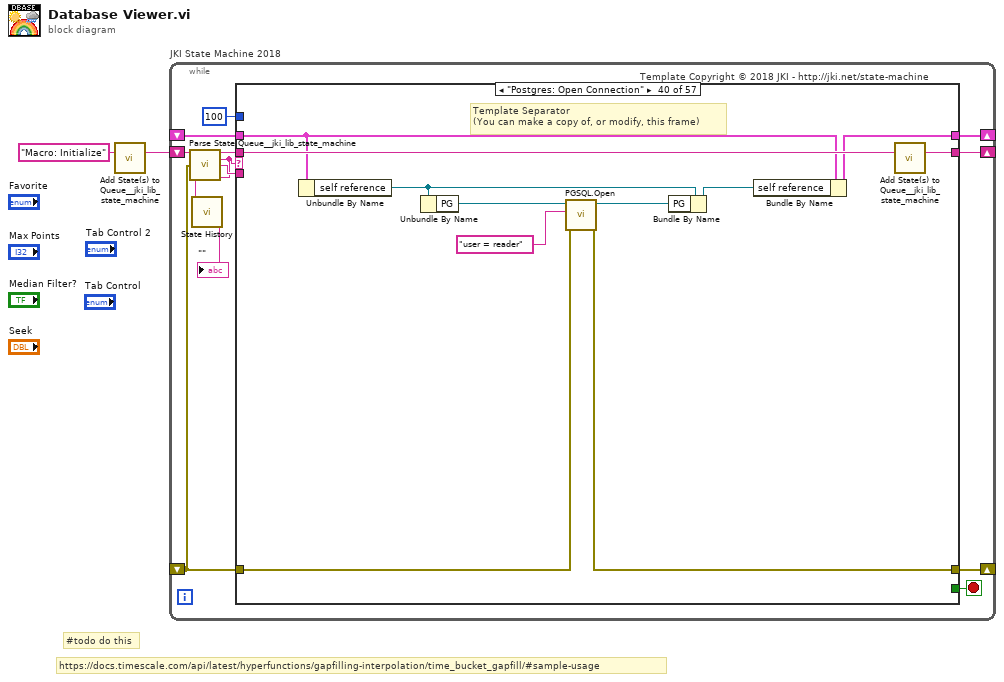
[diagram p0: block diagram]
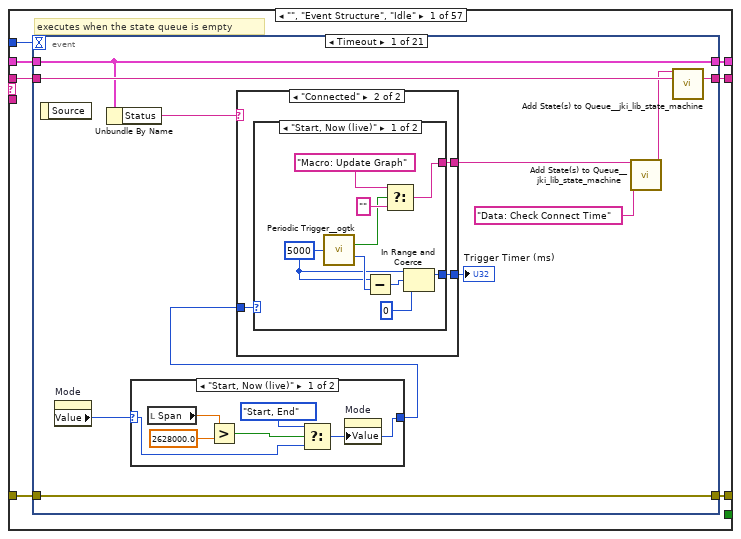
[diagram p2: hidden frame]
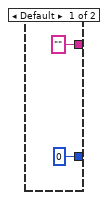
[diagram p4: hidden frame]
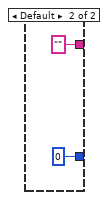
[diagram p5: hidden frame]
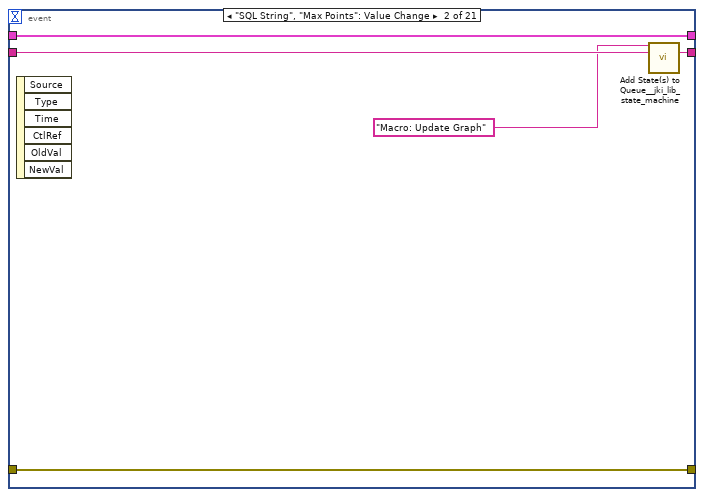
[diagram p6: hidden frame]
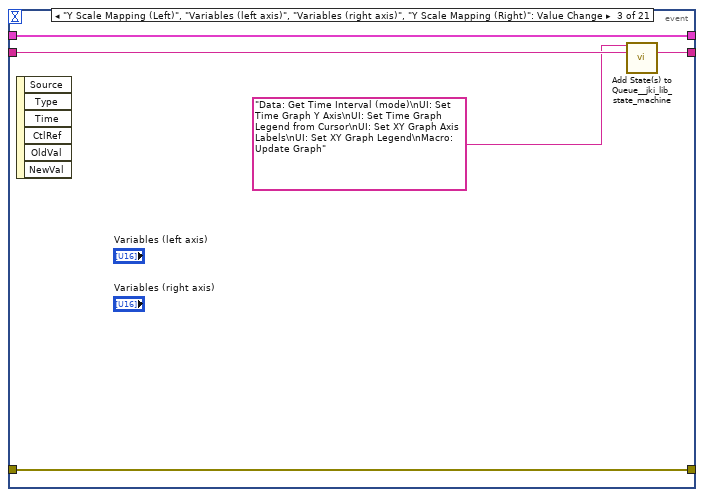
[diagram p7: hidden frame]
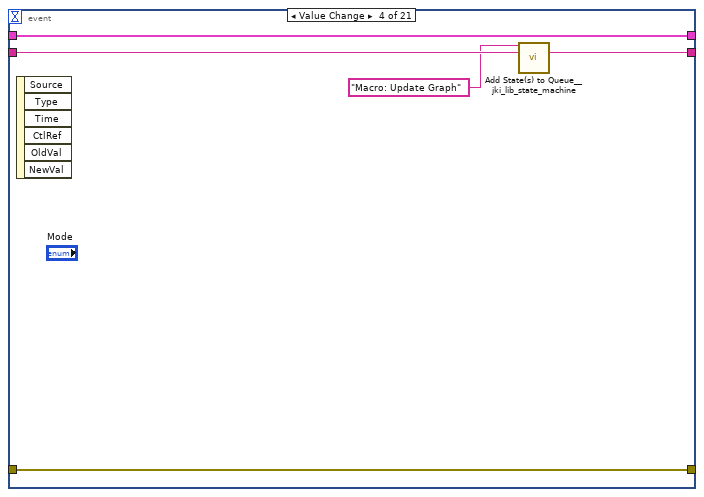
[diagram p8: hidden frame]
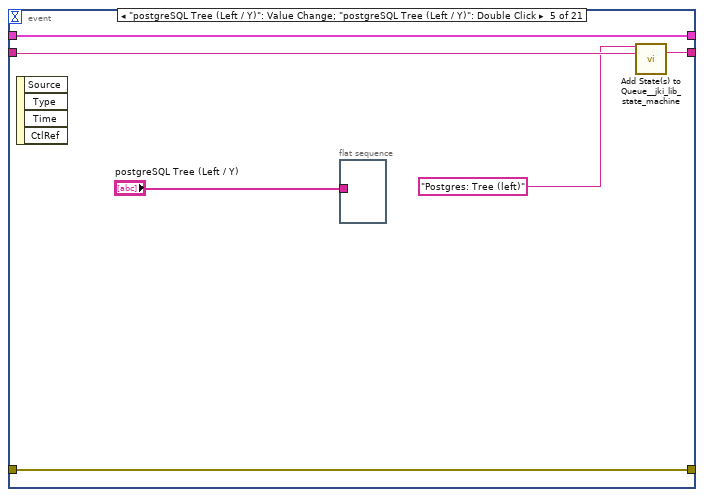
[diagram p9: hidden frame]
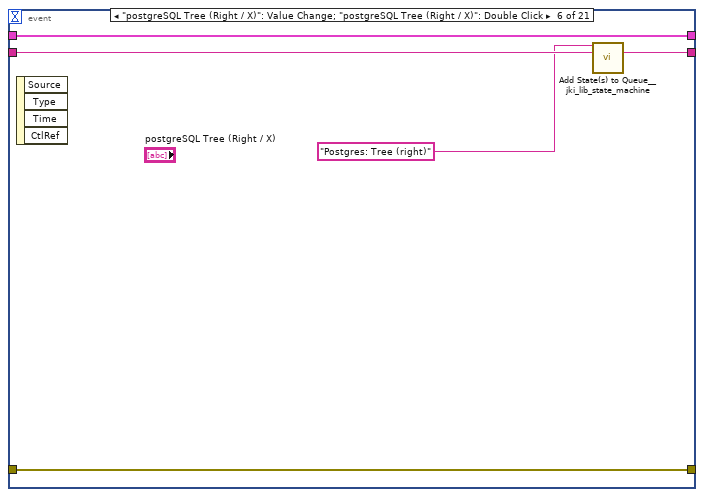
[diagram p10: hidden frame]
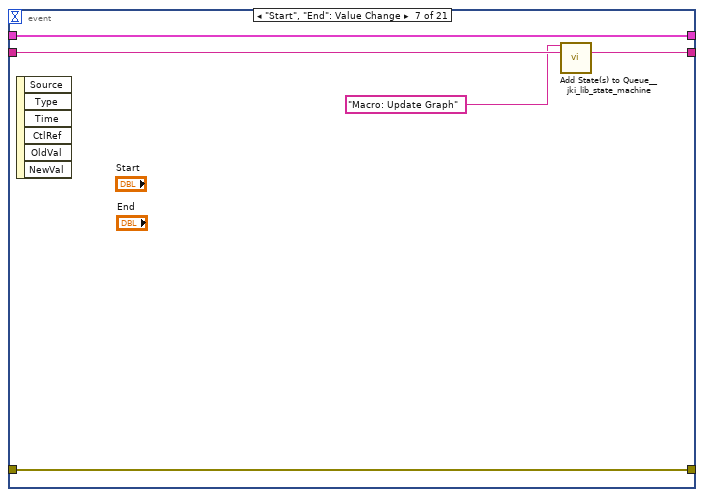
[diagram p11: hidden frame]
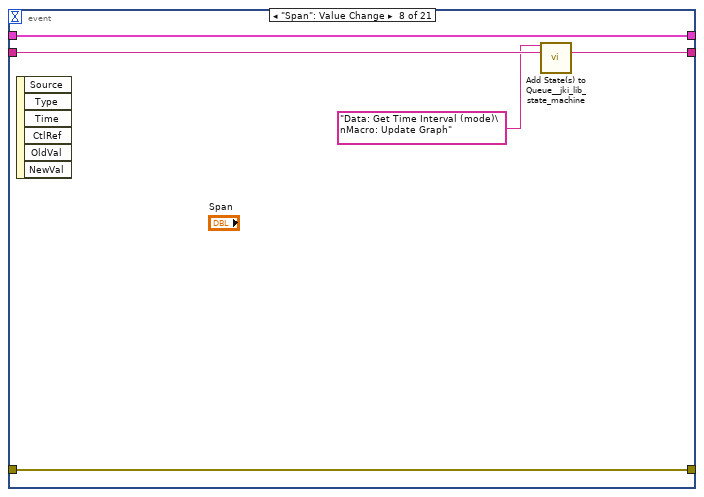
[diagram p12: hidden frame]
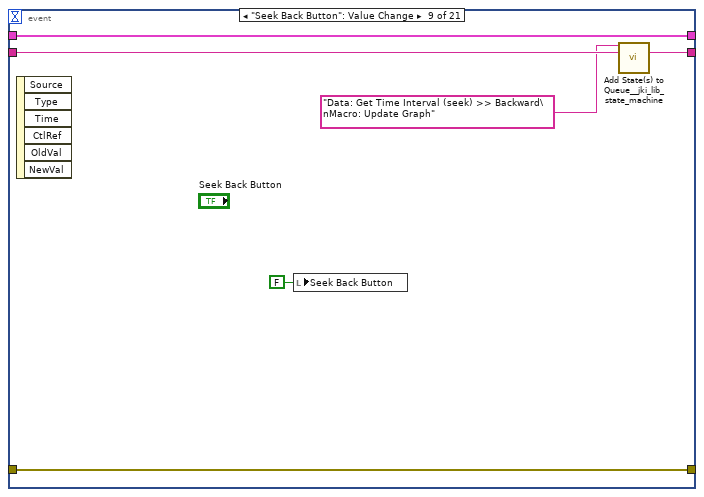
[diagram p13: hidden frame]
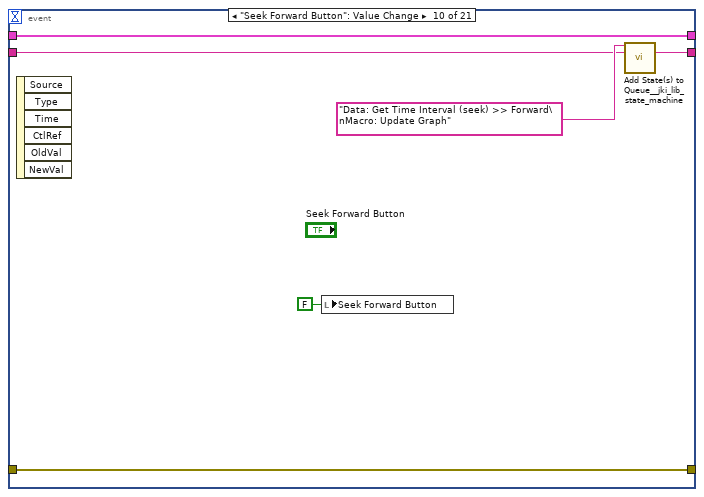
[diagram p14: hidden frame]
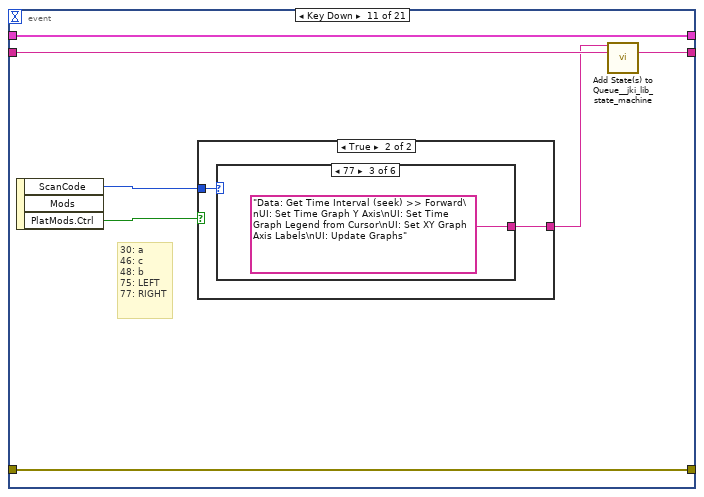
[diagram p15: hidden frame]
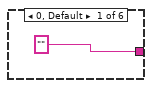
[diagram p17: hidden frame]
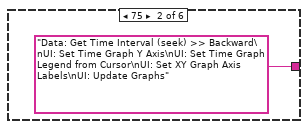
[diagram p18: hidden frame]
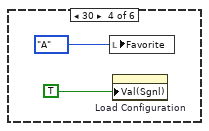
[diagram p19: hidden frame]
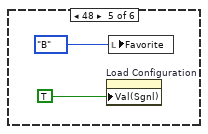
[diagram p20: hidden frame]
diagram:
  # "#todo do this"
  # "https://docs.timescale.com/api/latest/hyperfunctions/gapfilling-interpolation/time_bucket_gapfill/#sample-usage"
  n1 = call <vilib>:"Add State(s) to Queue__jki_lib_state_machine.vi"("State(s) in (\"\")"="Macro: Initialize") -> ("States Out"=w2:string)  [unwired: 14 in]
  n2 = while "JKI State Machine 2018" {
    shift-right: [w9] -> _
    shift-left: _ -> [w7]
    shift-right: [w11] -> _
    shift-left: _ -> [w6]
    shift-right: [w10] -> _
    shift-left: w2 -> [w12]
    stop <- w8 stop-if-true
    # "Template Copyright © 2018 JKI - http://jki.net/state-machine"
    n3 = call <vilib>:"Parse State Queue__jki_lib_state_machine.vi"("State Queue"=w12, "Error In (no error)"=w6) -> ("Remaining States"=w14:string, "Current State"=w4:string, "Arguments"=w13:string)  [unwired: 11 in]
    n4 = call <userlib>:"State History.vi"("Current State"=w4) -> ("History"=→"\"\"":string)  [unwired: 10 in]
    n5 = case shown="\"Postgres: Open Connection\"" w4 {
      selector: w4 -> [_ _ w196 _ _ _ _ _ _ _ _ _ _ _ _ _ _ _ _ _ _ _ _ _ _ _ _ _ _ _ _ _ _ _ _ _ _ _ _ _ _ _ _ _ _ _ _ _ _ _ _ _ _ _ _ _ _]
      tunnel: w14 -> [w21 w195 w200 w219 _ w229 w233 w254 w271 w300 w320 w335 w342 w351 w362 w366 w397 w403 w414 w484 w494 w526 w554 w579 w617 w631 w646 w671 w678 w689 w695 w700 w705 w710 w719 w728 w738 w749 w753 w764 w776 w790 w838 w849 w861 w876 w880 w908 w946 w959 w977 w992 w1008 w1020 w1029 w1051 w1067]
      tunnel: w13 -> [_ _ _ _ _ _ _ _ _ w296 _ _ w336 _ _ _ _ w398 w408 _ _ _ _ _ _ _ _ _ w674 w683 _ _ _ _ w713 w722 _ _ _ _ _ _ _ _ _ _ _ _ _ _ _ _ w993 _ _ _ _]
      tunnel: w7 -> [w19 w192 w198 w212 w222 w227 w230 _ w266 w295 w313 w332 w339 w348 w357 w363 w379 w401 w410 w481 w492 w523 w551 w576 w615 w628 w643 w667 w675 w685 w692 w697 w702 w707 w716 w725 w735 w746 w750 w761 w770 w780 w825 w843 w858 w871 w877 w903 w943 w955 w974 w989 w1006 w1017 w1022 w1048 w1060]
      tunnel: [w18 w193 w202 w216 errorcluster {"status"=FALSE, "code"=0, "source"=""} ("error out") w226 w231 w252 w262 w291 w318 w333 w340 w349 w358 w364 w369 w399 w411 w482 w489 w524 w541 w566 w609 w629 w642 w668 w676 w687 w693 w698 w703 w708 w717 w726 w736 w747 w751 w760 w771 w781 w824 w847 w859 w873 w878 w897 w940 w957 w970 w990 w1004 w1011 w1023 w1049 w1065] -> w11
      tunnel: w6 -> [w17 w193 w201 w216 w221 w226 w231 w252 w263 w292 w318 w333 w340 w349 w359 w364 w385 w400 w412 w482 w489 w524 w540 w565 w608 w629 w641 w669 w676 w687 w693 w698 w703 w708 w717 w726 w736 w747 w751 w755 w772 w782 w819 w847 w859 w874 w878 w894 w935 w957 w964 w990 w996 w1016 w1024 w1049 w1065]
      tunnel: [w20 w194 w199 w218 w224 w228 w232 w253 w270 w299 w319 w334 w341 w350 w361 w365 w396 w402 w413 w483 w493 w525 w553 w578 w616 w630 w645 w670 w677 w688 w694 w699 w704 w709 w718 w727 w737 w748 w752 w763 w775 w789 w837 w848 w860 w875 w879 w907 w945 w958 w976 w991 w1007 w1019 w1028 w1050 w1066] -> w10
      tunnel: [_ _ _ _ _ TRUE _ _ _ _ _ _ _ _ _ _ _ _ _ _ _ _ _ _ _ _ _ _ _ _ _ _ _ _ _ _ _ _ _ _ _ _ _ _ _ _ _ _ _ _ _ _ _ _ _ _ _] -> w8
      tunnel: [w16 w192 w198 w217 w222 w227 w230 w245 w269 w298 w314 w332 w338 w348 w357 w363 w379 w401 w410 w481 w492 w523 w551 w576 w615 w628 w643 w667 w675 w684 w692 w697 w702 w707 w716 w725 w735 w746 w750 w762 w774 w783 w826 w843 w858 w872 w877 w906 w944 w955 w974 w989 w1002 w1015 w1025 w1047 w1060] -> w9
      tunnel: 100 ("to") -> [w15 _ _ _ _ _ _ _ _ _ _ _ _ _ _ _ _ _ _ _ _ _ _ _ _ _ _ _ _ _ _ _ _ _ _ _ _ _ _ _ _ _ _ _ _ _ _ _ _ _ _ _ _ _ _ _ _]
      frame "", "Event Structure", "Idle" {
        # "executes when the state queue is empty"
        n6 = event shown="[0] Timeout" {
          selector: _ -> [_ _ _ _ _ _ _ _ _ _ _ _ _ _ _ _ _ _ _ _ _]
          dyn-events: _ -> [_ _ _ _ _ _ _ _ _ _ _ _ _ _ _ _ _ _ _ _ _]
          timeout: w15 -> [_ _ _ _ _ _ _ _ _ _ _ _ _ _ _ _ _ _ _ _ _]
          tunnel: w21 -> [w32 w60 w65 w67 w73 w81 w84 w89 w97 w101 w109 w126 w135 w140 w146 w152 w161 w169 w173 w181 w189]
          tunnel: [w31 w59 w64 w68 w74 w80 w85 w90 w96 w102 w110 w127 w136 w141 w147 w153 w160 w168 w174 w183 w191] -> w20
          tunnel: w19 -> [w26 w57 w61 w70 w75 w79 w86 w91 w94 w99 w104 w128 w137 w142 w148 w154 w162 w170 w175 w178 w186]
          tunnel: [w30 w58 w62 w69 w76 w78 w83 w88 w95 w100 w105 w123 w133 w138 w144 w150 w159 w167 w171 w182 w190] -> w18
          tunnel: w17 -> [w30 w58 w62 w69 w76 w78 w83 w88 w95 w100 w105 w123 w133 w138 w144 w150 w159 w167 w171 w182 w190]
          tunnel: [w26 w57 w61 w70 w75 w79 w86 w91 w94 w99 w104 w124 w137 w142 w148 w154 w162 w170 w175 w177 w185] -> w16
          event Timeout {
            n7 = event-data() -> ()  [unwired: 1 in, 1 out]
            n8 = property on="Mode" class="Enum (strict)"() -> ("Value"=w23:T2)  [unwired: 2 in, 2 out]
            n9 = Unbundle By Name(w26) -> ("Status"=w24:string)
            n10 = case shown="\"Start, Now (live)\"" w23 {
              selector: w23 -> [w35 w39]
              tunnel: [w33 w39] -> w22
              frame "Start, Now (live)" {
                n11 = local read "Span"() -> (w38:dbl)
                n12 = Greater?(x=w38, y=2628000.0) -> (0:w36:bool)
                n13 = Select(t=Time_Mode--enum."Start, End" ("Mode"), s=w36, f=w35) -> (s? t:f=w33:T2)
                n14 = property on="Mode" class="Enum (strict)"("Value"=w33) -> ()  [unwired: 2 in, 2 out]
              }
              frame Default {
              }
            }
            n15 = case shown="\"Connected\"" w24 {
              tunnel: [u32 0 ("time (ms)") w44] -> w27
              tunnel: ["" ("f") w43] -> w25
              tunnel: w22 -> [_ w42]
              frame Default {
              }
              frame "Connected" {
                n16 = case shown="\"Start, Now (live)\"" w42 {
                  tunnel: [w52 "" ("f")] -> w43
                  tunnel: [w45 u32 0 ("time (ms)")] -> w44
                  frame "Start, Now (live)" {
                    w47 = u32 5000 ("time (ms)")
                    n17 = call <userlib>:"Periodic Trigger__ogtk.vi"("time (ms)"=w47) -> ("Triggered"=w50:bool, "timer value"=w49:u32)  [unwired: 12 in, 1 out]
                    n18 = Subtract(x=w47, y=w49) -> (x-y=w48:u32)
                    n19 = Select(t="Macro: Update Graph" ("State(s) in Front (\"\")"), s=w50, f="") -> (s? t:f=w52:string)
                    n20 = In Range and Coerce(upper limit=w47, x=w48, lower limit=u32 0) -> (coerced(x)=w45:u32)  [unwired: 1 out]
                  }
                  frame Default {
                  }
                }
              }
            }
            "Trigger Timer (ms)" <- w27
            n21 = call <vilib>:"Add State(s) to Queue__jki_lib_state_machine.vi"("State(s) in Front (\"\")"=w25, "State(s) at Back (\"\")"="Data: Check Connect Time" ("State(s) in Front (\"\")")) -> ("States Out"=w28:string)  [unwired: 13 in]
            n22 = call <vilib>:"Add State(s) to Queue__jki_lib_state_machine.vi"("State(s) in Front (\"\")"=w28, "State(s) in (\"\")"=w32) -> ("States Out"=w31:string)  [unwired: 13 in]
          }
          event "SQL String", "Max Points": Value Change {
            n23 = event-data() -> ()  [unwired: 1 in, 6 out]
            n24 = call <vilib>:"Add State(s) to Queue__jki_lib_state_machine.vi"("State(s) in Front (\"\")"="Macro: Update Graph" ("State(s) in Front (\"\")"), "State(s) in (\"\")"=w60) -> ("States Out"=w59:string)  [unwired: 13 in]
          }
          event "Y Scale Mapping (Left)", "Variables (left axis)", "Variables (right axis)", "Y Scale Mapping (Right)": Value Change {
            n25 = event-data() -> ()  [unwired: 1 in, 6 out]
            n26 = call <vilib>:"Add State(s) to Queue__jki_lib_state_machine.vi"("State(s) in Front (\"\")"="Data: Get Time Interval (mode)\nUI: Set Time Graph Y Axis\nUI: Set Time Graph Legend from Cursor\nUI: Set XY Graph Axis Labels\nUI: Set XY Graph Legend\nMacro: Update Graph" ("State(s) in Front (\"\")"), "State(s) in (\"\")"=w65) -> ("States Out"=w64:string)  [unwired: 13 in]
          }
          event Value Change {
            n27 = event-data() -> ()  [unwired: 1 in, 6 out]
            n28 = call <vilib>:"Add State(s) to Queue__jki_lib_state_machine.vi"("State(s) in Front (\"\")"="Macro: Update Graph" ("State(s) in Front (\"\")"), "State(s) in (\"\")"=w67) -> ("States Out"=w68:string)  [unwired: 13 in]
          }
          event "postgreSQL Tree (Left / Y)": Value Change; "postgreSQL Tree (Left / Y)": Double Click {
            n29 = event-data() -> ()  [unwired: 1 in, 4 out]
            n30 = flat-sequence {
              tunnel: "postgreSQL Tree (Left / Y)" -> [_]
              frame #0 {
              }
            }
            n31 = call <vilib>:"Add State(s) to Queue__jki_lib_state_machine.vi"("State(s) in Front (\"\")"="Postgres: Tree (left)" ("State(s) in Front (\"\")"), "State(s) in (\"\")"=w73) -> ("States Out"=w74:string)  [unwired: 13 in]
          }
          event "postgreSQL Tree (Right / X)": Value Change; "postgreSQL Tree (Right / X)": Double Click {
            n32 = event-data() -> ()  [unwired: 1 in, 4 out]
            n33 = call <vilib>:"Add State(s) to Queue__jki_lib_state_machine.vi"("State(s) in Front (\"\")"="Postgres: Tree (right)" ("State(s) in Front (\"\")"), "State(s) in (\"\")"=w81) -> ("States Out"=w80:string)  [unwired: 13 in]
          }
          event "Start", "End": Value Change {
            n34 = event-data() -> ()  [unwired: 1 in, 6 out]
            n35 = call <vilib>:"Add State(s) to Queue__jki_lib_state_machine.vi"("State(s) in Front (\"\")"="Macro: Update Graph" ("State(s) in Front (\"\")"), "State(s) in (\"\")"=w84) -> ("States Out"=w85:string)  [unwired: 13 in]
          }
          event "Span": Value Change {
            n36 = event-data() -> ()  [unwired: 1 in, 6 out]
            n37 = call <vilib>:"Add State(s) to Queue__jki_lib_state_machine.vi"("State(s) in Front (\"\")"="Data: Get Time Interval (mode)\nMacro: Update Graph" ("State(s) in Front (\"\")"), "State(s) in (\"\")"=w89) -> ("States Out"=w90:string)  [unwired: 13 in]
          }
          event "Seek Back Button": Value Change {
            n38 = event-data() -> ()  [unwired: 1 in, 6 out]
            n39 = local write "Seek Back Button"(FALSE ("Seek Back Button")) -> ()
            n40 = call <vilib>:"Add State(s) to Queue__jki_lib_state_machine.vi"("State(s) in Front (\"\")"="Data: Get Time Interval (seek) >> Backward\nMacro: Update Graph" ("State(s) in Front (\"\")"), "State(s) in (\"\")"=w97) -> ("States Out"=w96:string)  [unwired: 13 in]
          }
          event "Seek Forward Button": Value Change {
            n41 = event-data() -> ()  [unwired: 1 in, 6 out]
            n42 = local write "Seek Forward Button"(FALSE ("Seek Forward Button")) -> ()
            n43 = call <vilib>:"Add State(s) to Queue__jki_lib_state_machine.vi"("State(s) in Front (\"\")"="Data: Get Time Interval (seek) >> Forward\nMacro: Update Graph" ("State(s) in Front (\"\")"), "State(s) in (\"\")"=w101) -> ("States Out"=w102:string)  [unwired: 13 in]
          }
          event Key Down {
            # "30: a\n46: c\n48: b\n75: LEFT\n77: RIGHT"
            n44 = event-data() -> ("ScanCode"=w107:i16, "PlatMods.Ctrl"=w108:bool)  [unwired: 1 in, 1 out]
            n45 = case shown="True" w108 {
              tunnel: w107 -> [_ w112]
              tunnel: [_ w111] -> w106
              frame False {
              }
              frame True {
                n46 = case shown="77" w112 {
                  tunnel: ["" ("State(s) in Front (\"\")") "Data: Get Time Interval (seek) >> Backward\nUI: Set Time Graph Y Axis\nUI: Set Time Graph Legend from Cursor\nUI: Set XY Graph Axis Labels\nUI: Update Graphs" ("State(s) in Front (\"\")") "Data: Get Time Interval (seek) >> Forward\nUI: Set Time Graph Y Axis\nUI: Set Time Graph Legend from Cursor\nUI: Set XY Graph Axis Labels\nUI: Update Graphs" ("State(s) in Front (\"\")") _ _ _] -> w111
                  frame 0, Default {
                  }
                  frame 75 {
                  }
                  frame 77 {
                  }
                  frame 30 {
                    n47 = local write "Favorite"(enum16{"A", "B", "C"}."A" ("Favorite")) -> ()
                    n48 = property on="Load Configuration" class="Bool (strict)"("Val(Sgnl)"=TRUE) -> ()  [unwired: 2 in, 2 out]
                  }
                  frame 48 {
                    n49 = property on="Load Configuration" class="Bool (strict)"("Val(Sgnl)"=TRUE) -> ()  [unwired: 2 in, 2 out]
                    n50 = local write "Favorite"(enum16{"A", "B", "C"}."B" ("Favorite")) -> ()
                  }
                  frame 46 {
                    n51 = local write "Favorite"(enum16{"A", "B", "C"}."C" ("Favorite")) -> ()
                    n52 = property on="Load Configuration" class="Bool (strict)"("Val(Sgnl)"=TRUE) -> ()  [unwired: 2 in, 2 out]
                  }
                }
              }
            }
            n53 = call <vilib>:"Add State(s) to Queue__jki_lib_state_machine.vi"("State(s) in Front (\"\")"=w106, "State(s) in (\"\")"=w109) -> ("States Out"=w110:string)  [unwired: 13 in]
          }
          event "Database Time Graph": Scale Range Change {
            n54 = event-data() -> ("NewRange"=w122:T9, "Kind"=w129:enum16{"X-Scale", "Y-Scale", "Z-Scale"})  [unwired: 1 in]
            n55 = case shown="\"X-Scale\", Default" w129 {
              tunnel: ["Database: Database Trace" ("State(s) in Front (\"\")") "" ("State(s) in Front (\"\")")] -> w125
              frame "X-Scale", Default {
              }
              frame "Y-Scale" {
              }
            }
            n56 = Bundle By Name(cluster=w128, "NewRange"=w122) -> (w124:T10)
            n57 = call <vilib>:"Add State(s) to Queue__jki_lib_state_machine.vi"("State(s) in Front (\"\")"=w125, "State(s) in (\"\")"=w126) -> ("States Out"=w127:string)  [unwired: 13 in]
          }
          event "Export Button": Value Change {
            n58 = event-data() -> ()  [unwired: 1 in, 6 out]
            n59 = local write "Export Button"(FALSE ("Export Button")) -> ()
            n60 = call <vilib>:"Add State(s) to Queue__jki_lib_state_machine.vi"("State(s) in Front (\"\")"="Data: Calculate Shift Hours\nDatabase: Export" ("State(s) in Front (\"\")"), "State(s) in (\"\")"=w135) -> ("States Out"=w136:string)  [unwired: 13 in]
          }
          event Panel Close? {
            n61 = event-data() -> ()  [unwired: 1 in, 4 out]
            n62 = call <vilib>:"Add State(s) to Queue__jki_lib_state_machine.vi"("State(s) in Front (\"\")"="Macro: Exit" ("State(s) in Front (\"\")"), "State(s) in (\"\")"=w140) -> ("States Out"=w141:string)  [unwired: 13 in]
            n63 = event-data("Discard?"=TRUE) -> ()  [unwired: 1 in, 1 out]
          }
          event "Igor", "DST": Value Change {
            n64 = event-data() -> ()  [unwired: 1 in, 6 out]
            n65 = call <vilib>:"Add State(s) to Queue__jki_lib_state_machine.vi"("State(s) in Front (\"\")"="Data: Calculate Shift Hours" ("State(s) in Front (\"\")"), "State(s) in (\"\")"=w146) -> ("States Out"=w147:string)  [unwired: 13 in]
          }
          event "Exit": Value Change {
            n66 = event-data() -> ()  [unwired: 1 in, 6 out]
            n67 = local write "Exit"(FALSE ("Exit")) -> ()
            n68 = call <vilib>:"Add State(s) to Queue__jki_lib_state_machine.vi"("State(s) in Front (\"\")"="Macro: Exit" ("State(s) in Front (\"\")"), "State(s) in (\"\")"=w152) -> ("States Out"=w153:string)  [unwired: 13 in]
          }
          event "Save Configuration": Value Change {
            n69 = event-data() -> ()  [unwired: 1 in, 6 out]
            n70 = local write "Save Configuration"(FALSE ("Save Configuration")) -> ()
            n71 = property on="Favorite" class="Enum (strict)"() -> ("RingText.Text"=w155:string)  [unwired: 2 in, 2 out]
            n72 = call <vilib>:"Build State String with Arguments__JKI_lib_State_Machine.vi"("Arguments (\"\")"=w155, "State"="Macro: Save Config" ("State(s) in Front (\"\")")) -> ("State with Arguments"=w156:string)  [unwired: 4 in]
            n73 = call <vilib>:"Add State(s) to Queue__jki_lib_state_machine.vi"("State(s) in Front (\"\")"=w156, "State(s) in (\"\")"=w161) -> ("States Out"=w160:string)  [unwired: 13 in]
          }
          event "Load Configuration": Value Change {
            n74 = event-data() -> ()  [unwired: 1 in, 6 out]
            n75 = local write "Load Configuration"(FALSE ("Load Configuration")) -> ()
            n76 = property on="Favorite" class="Enum (strict)"() -> ("RingText.Text"=w165:string)  [unwired: 2 in, 2 out]
            n77 = call <vilib>:"Build State String with Arguments__JKI_lib_State_Machine.vi"("Arguments (\"\")"=w165, "State"="Macro: Load Config" ("State(s) in Front (\"\")")) -> ("State with Arguments"=w163:string)  [unwired: 4 in]
            n78 = call <vilib>:"Add State(s) to Queue__jki_lib_state_machine.vi"("State(s) in Front (\"\")"=w163, "State(s) in (\"\")"=w169) -> ("States Out"=w168:string)  [unwired: 13 in]
          }
          event "Trees Visible? >>>>>>": Value Change {
            n79 = event-data() -> ()  [unwired: 1 in, 6 out]
            n80 = call <vilib>:"Add State(s) to Queue__jki_lib_state_machine.vi"("State(s) in Front (\"\")"="UI: Hide/show trees" ("State(s) in Front (\"\")"), "State(s) in (\"\")"=w173) -> ("States Out"=w174:string)  [unwired: 13 in]
          }
          event "Connect": Value Change {
            w179 = string[] [] ("Variable Names")
            n81 = event-data() -> ()  [unwired: 1 in, 6 out]
            n82 = local write "Connect"(FALSE ("Connect")) -> ()
            n83 = Bundle By Name(cluster=w178, "Variable Names"=w179, "Variable Paths"=w179) -> (w177:T10)
            n84 = call <vilib>:"Add State(s) to Queue__jki_lib_state_machine.vi"("State(s) in Front (\"\")"="Macro: Connect", "State(s) in (\"\")"=w181) -> ("States Out"=w183:string)  [unwired: 13 in]
          }
          event "Disconnect": Value Change {
            w187 = string[] [] ("Variable Names")
            n85 = event-data() -> ()  [unwired: 1 in, 6 out]
            n86 = local write "Disconnect"(FALSE ("Connect")) -> ()
            n87 = Bundle By Name(cluster=w186, "Variable Names"=w187, "Variable Paths"=w187) -> (w185:T10)
            n88 = call <vilib>:"Add State(s) to Queue__jki_lib_state_machine.vi"("State(s) in Front (\"\")"="Macro: Disconnect", "State(s) in (\"\")"=w189) -> ("States Out"=w191:string)  [unwired: 13 in]
          }
        }
      }
      frame "---------- Core ----------" {
        # "Do not put any code in this frame.\n(it is a separator no-op)"
        n89 = call <vilib>:"Add State(s) to Queue__jki_lib_state_machine.vi"("State(s) in (\"\")"=w195) -> ("States Out"=w194:string)  [unwired: 14 in]
      }
      frame Default {
        w205 = 42 items=["No error", "Argument error", "Memory is full", "Out of zone", "End of file", "File already open", "Generic file I/O error", "File not found", "File permission error", "Disk is full", "Duplicate path", "Too many files open", "System feature not enabled", "Resource file not found", "Cannot add resource", "Resource not found", "Image not found", "Image memory error", "Pen does not exist", "Config type invalid", "Config token not found", "Config parse error", "Config memory error", "Bad external code format", "Bad external code offset", "External code not present", "Null window", "Destroy window error", "Null menu", "Print aborted", "Bad print record", "Print driver error", "Windows error during printing", "Memory error during printing", "Print dialog error", "Generic print error", "Invalid device refnum", "Device not found", "Device parameter error", "Device unit error", "Cannot open device", "Device call aborted", "Generic error", "Cancelled by user", "Object ID too low", "Object ID too high", "Object not in heap", "Unknown heap", "Unknown object (invalid DefProc)", "Unknown object (DefProc not in table)", "Message out of range", "Invalid (null) method", "Unknown message", "Manager call not supported", "Bad address", "Network operation in progress", "Network operation timed out", "Connection is busy", "Network attribute not supported", "Network error", "Address in use", "System out of memory", "Connection aborted", "Connection refused", "Not connected", "Already connected", "Connection closed", "Initialization error (interapplication manager)", "Bad occurrence", "Wait on unbound occurrence handler", "Occurrence queue overflow", "Datalog type conflict", "Unused", "Unrecognized type (interapplication manager)", "Memory corrupt", "Failed to make temporary DLL", "Old CIN version", "Drag socket not found", "Failed to load drop-object", "Failed to register OLE object", "Failed to release OLE object", "Format specifier type mismatch", "Unknown format specifier", "Too few format specifiers", "Too many format specifiers", "Scan failed", "Newer CIN version", "Error converting to variant", "Runtime menu error", "Password tampered", "Variant attribute not found", "Incompatible variant data type", "Event data is not available", "Event Store is not present", "Occurrence is not found", "Event Queue is not created", "Event info is not available", "Refnum passed is NULL", "Error retrieving Class GUID", "Error retrieving CoClass GUID", "Error retrieving TypeLib GUID.", "Bad built application magic bytes.", "Specific driver is different from the specific driver associated with the Logical Name.", "There is no session opened to the class driver.", "Max Error", "MAX - Error with config objects", "MAX - Error loading configuration", "MAX - Group not supported"]
        # "Current State"
        # "Do not delete, rename, or modify this frame.\n(this is used to capture unhandled states and typos)"
        # "Handle mistyped state name (developer tool)"
        n90 = Format Into String(format string="Software Exception: Unhandled State \"%s\"." ("message"), error in=w201, w196) -> (resulting string=w204:string, error out=w203:errorcluster)  [unwired: 1 in]
        n91 = call <vilib>:"Error Cluster From Error Code.vi"("show call chain? (False)"=TRUE, "error in (no error)"=w203, "error message (\"\")"=w204, "error code (0)"=w205) -> ("error out"=w202:errorcluster)  [unwired: 5 in]
        n92 = call <vilib>:"Add State(s) to Queue__jki_lib_state_machine.vi"("State(s) in (\"\")"=w200) -> ("States Out"=w199:string)  [unwired: 14 in]
      }
      frame "Initialize Core Data" {
        # "Do not delete, rename, or modify this frame.\n(this is used to determine panel behavior on exit)"
        # "originally closed?"
        # "exe?"
        # "If panel starts closed or is an EXE, then close it when we exit"
        n93 = property class="VI"() -> ("FP.State"=w209:T5)  [unwired: 2 in, 2 out]
        n94 = property class="App"() -> ("App.Kind"=w215:T6)  [unwired: 2 in, 2 out]
        n95 = control-ref of="Current VI Reference"() -> (w210:refnum<vi>)
        n96 = Equal?(x=w209, y=T5."Closed" ("Front Panel Window:State")) -> (x = y?=w207:bool)
        n97 = Equal?(x=w215, y=T6."Run Time System" ("Application:Kind")) -> (x = y?=w213:bool)
        n98 = Or(x=w207, y=w213) -> (x .or. y?=w211:bool)
        n99 = Bundle By Name(cluster=w212, "Core.Current VI Reference"=w210, "Core.Close Panel on Exit?"=w211) -> (w217:T10)
        n100 = call <vilib>:"Add State(s) to Queue__jki_lib_state_machine.vi"("State(s) in (\"\")"=w219) -> ("States Out"=w218:string)  [unwired: 14 in]
      }
      frame "Error Handler" {
        # "clear the queue if there is an error"
        # "Unhandled Error -- Display it"
        # "Handle any errors here.\nYou can also output any states to clean-up after errors occur"
        # "Clear error"
        n101 = call <vilib>:"General Error Handler.vi"("error in (no error)"=w221) -> ()  [unwired: 10 in, 5 out]
        n102 = call <vilib>:"Add State(s) to Queue__jki_lib_state_machine.vi"("State(s) in Front (\"\")"="/* Post Error States") -> ("States Out"=w224:string)  [unwired: 14 in]
      }
      frame "Exit" {
        # "Do not put any code in this frame.\n(No errors that occur here will be handled.)"
        n103 = call <vilib>:"Add State(s) to Queue__jki_lib_state_machine.vi"("State(s) in (\"\")"=w229) -> ("States Out"=w228:string)  [unwired: 14 in]
      }
      frame "---------- Data ----------" {
        # "Do not put any code in this frame.\n(It is a separator no-op. You can make a copy of this frame to create a new Data frame)"
        n104 = call <vilib>:"Add State(s) to Queue__jki_lib_state_machine.vi"("State(s) in (\"\")"=w233) -> ("States Out"=w232:string)  [unwired: 14 in]
      }
      frame "Data: Initialize" {
        w234 = ""  # Status
        w235 = timestamp(0 s since 1904-01-01)  # Connect Time
        w238 = refnum<class "Database Viewer.lvclass"> refnum  # self reference
        w240 = T8 {"Variables (left axis)"=[], "Variables (right axis)"=[], "Time Mode"=enum."Start + Span", "Time Bucket"=enum."max points", "Start Time"=timestamp(0 s since 1904-01-01), "End Time"=timestamp(0 s since 1904-01-01), "Step Size"=0.0, "Y Scale Mapping (left)"=enum."linear", "max points per trace (all)"=0, "Y Scale Mapping (right)"=enum."linear", "Filter?"=FALSE, "export path"=path "", "DST"=FALSE}  # Controls Cluster
        w237 = refnum<class "Configuration.lvclass"> refnum  # Configuration
        w241 = 0  # No. of non PG vars
        w242 = T11 {"Table Names"=[], "Table Paths"=[], "PG Columns"=[], "Columns (right)"=[], "PG Names"=[]}  # PG Variables
        w243 = cluster{string, i32}[] []  # Ring items
        w246 = T12 {"start timestamp"=timestamp(0 s since 1904-01-01), "stop timestamp (now)"=timestamp(0 s since 1904-01-01)}  # Time Interval
        w249 = string[] []  # Variable Paths
        w236 = path ""  # Database
        w250 = string[] []  # Variable Names
        w248 = T9 {"Minimum"=0.0, "Maximum"=0.0, "Increment"=0.0, "Minor Increment"=0.0, "Start"=0.0}  # NewRange
        w244 = T4 []  # Traces
        w251 = T13 {"Current VI Reference"=refnum, "Close Panel on Exit?"=FALSE}  # Core
        # "Initialize the shift-register data, here.\n(data names are defined by what you wire into the bundle function)"
        n105 = control-ref of="XY Graph"() -> (w239:refnum<vi>)
        n106 = control-ref of="Time Graph"() -> (w247:refnum<vi>)
        n107 = call <vilib>:"Add State(s) to Queue__jki_lib_state_machine.vi"("State(s) in (\"\")"=w254) -> ("States Out"=w253:string)  [unwired: 14 in]
        n108 = Bundle("Core"=w251, "self reference"=w238, "Configuration"=w237, "Database"=w236, "Connect Time"=w235, "Variable Names"=w250, "Variable Paths"=w249, "Traces"=w244, "NewRange"=w248, "Time Graph"=w247, "XY Graph"=w239, "Time Interval"=w246, "Ring items"=w243, "PG Variables"=w242, "No. of non PG vars"=w241, "Controls Cluster"=w240, "Status"=w234) -> (w245:T10)  [unwired: 1 in]
      }
      frame "Data: Get Time Interval (mode)" {
        # "update time interval cluster\n& calculate span"
        # "refresh x axis range"
        # "write to FP controls"
        # "calculate new start or end times"
        # "Do not put any code in this frame.\n(It is a separator no-op. You can make a copy of this frame to create a new Data frame)"
        n109 = property on="Mode" class="Enum (strict)"() -> ("Value"=w268:T2)  [unwired: 2 in, 2 out]
        n110 = Unbundle By Name(w266) -> ("Time Graph"=w267:refnum<vi>)
        n111 = case shown="\"Start, Now (live)\"" w268 {
          tunnel: [w272 w275 w278 w282] -> w265
          tunnel: [w273 w276 w277 w281] -> w264
          frame "Start, Now (live)" {
            n112 = property on="Start" class="DigNum (strict)"() -> ("Value"=w273:dbl)  [unwired: 2 in, 2 out]
            n113 = Get Date/Time In Seconds() -> (seconds since 1Jan1904=w274:timestamp)
            n114 = To Double Precision Float(number=w274) -> (double precision float=w272:dbl)
          }
          frame "Start, End" {
            n115 = property on="Start" class="DigNum (strict)"() -> ("Value"=w276:dbl)  [unwired: 2 in, 2 out]
            n116 = property on="End" class="DigNum (strict)"() -> ("Value"=w275:dbl)  [unwired: 2 in, 2 out]
          }
          frame "Start + Span" {
            n117 = property on="Start" class="DigNum (strict)"() -> ("Value"=w277:dbl)  [unwired: 2 in, 2 out]
            n118 = property on="Span" class="DigNum (strict)"() -> ("Value"=w279:dbl)  [unwired: 2 in, 2 out]
            n119 = Add(x=w277, y=w279) -> (x+y=w278:dbl)
          }
          frame "End - Span" {
            n120 = property on="Start" class="DigNum (strict)"() -> ("Value"=w281:dbl)  [unwired: 2 in, 2 out]
            n121 = property on="Span" class="DigNum (strict)"() -> ("Value"=w283:dbl)  [unwired: 2 in, 2 out]
            n122 = property on="End" class="DigNum (strict)"() -> ("Value"=w280:dbl)  [unwired: 2 in, 2 out]
            n123 = Subtract(x=w280, y=w283) -> (x-y=w282:dbl)
          }
        }
        n124 = property on="Start" class="DigNum (strict)"("Value"=w264) -> ()  [unwired: 2 in, 2 out]
        n125 = property on="End" class="DigNum (strict)"("Value"=w265) -> ()  [unwired: 2 in, 2 out]
        n126 = local read "Time Bucket"() -> (w255:T1)
        n127 = To Time Stamp(1:w265) -> (0:w261:timestamp)
        n128 = To Time Stamp(1:w264) -> (0:w260:timestamp)
        n129 = call "Set Time Graph X Axis.vi"("error in (no error)"=w263, "End"=w261, "Start"=w260, "reference in"=w267) -> ("error out"=w262:errorcluster)  [unwired: 6 in, 1 out]
        n130 = call "Convert Times to Interval and Span.vi"("Time Bucket"=w255, "End"=w261, "Start"=w260) -> ("Time Bucket out"=w256:T1, "Span"=w259:dbl, "time interval"=w258:T12)  [unwired: 6 in]
        n131 = Bundle By Name(cluster=w266, "Time Interval"=w258) -> (w269:T10)
        n132 = local write "Time Bucket"(w256) -> ()
        n133 = property on="Span" class="DigNum (strict)"("Value"=w259) -> ()  [unwired: 2 in, 2 out]
        n134 = call <vilib>:"Add State(s) to Queue__jki_lib_state_machine.vi"("State(s) in Front (\"\")"="Data: Write Time Interval" ("State(s) in Front (\"\")"), "State(s) in (\"\")"=w271) -> ("States Out"=w270:string)  [unwired: 13 in]
      }
      frame "Data: Get Time Interval (seek)" {
        # "update time interval cluster\n& calculate span"
        # "refresh x axis range"
        # "write to FP controls"
        # "calculate new start or end times"
        # "Do not put any code in this frame.\n(It is a separator no-op. You can make a copy of this frame to create a new Data frame)"
        n135 = case shown="\"Forward\", Default" w296 {
          tunnel: [w301 w308] -> w293
          tunnel: [w302 w309] -> w294
          frame "Backward" {
            n136 = property on="Start" class="DigNum (strict)"() -> ("Value"=w303:dbl)  [unwired: 2 in, 2 out]
            n137 = property on="Seek" class="DigNum (strict)"() -> ("Value"=w305:dbl)  [unwired: 2 in, 2 out]
            n138 = property on="End" class="DigNum (strict)"() -> ("Value"=w304:dbl)  [unwired: 2 in, 2 out]
            n139 = property on="Seek" class="DigNum (strict)"() -> ("Value"=w306:dbl)  [unwired: 2 in, 2 out]
            n140 = Subtract(x=w303, y=w305) -> (x-y=w302:dbl)
            n141 = Subtract(x=w304, y=w306) -> (x-y=w301:dbl)
          }
          frame "Forward", Default {
            n142 = property on="Start" class="DigNum (strict)"() -> ("Value"=w310:dbl)  [unwired: 2 in, 2 out]
            n143 = property on="Seek" class="DigNum (strict)"() -> ("Value"=w312:dbl)  [unwired: 2 in, 2 out]
            n144 = property on="End" class="DigNum (strict)"() -> ("Value"=w311:dbl)  [unwired: 2 in, 2 out]
            n145 = property on="Seek" class="DigNum (strict)"() -> ("Value"=w307:dbl)  [unwired: 2 in, 2 out]
            n146 = Add(x=w311, y=w307) -> (x+y=w308:dbl)
            n147 = Add(x=w310, y=w312) -> (x+y=w309:dbl)
          }
        }
        n148 = property on="Start" class="DigNum (strict)"("Value"=w294) -> ()  [unwired: 2 in, 2 out]
        n149 = property on="End" class="DigNum (strict)"("Value"=w293) -> ()  [unwired: 2 in, 2 out]
        n150 = To Time Stamp(1:w294) -> (0:w290:timestamp)
        n151 = To Time Stamp(1:w293) -> (0:w289:timestamp)
        n152 = Unbundle By Name(w295) -> ("Time Graph"=w297:refnum<vi>)
        n153 = local read "Time Bucket"() -> (w284:T1)
        n154 = call "Set Time Graph X Axis.vi"("error in (no error)"=w292, "End"=w289, "Start"=w290, "reference in"=w297) -> ("error out"=w291:errorcluster)  [unwired: 6 in, 1 out]
        n155 = call "Convert Times to Interval and Span.vi"("Time Bucket"=w284, "End"=w289, "Start"=w290) -> ("Time Bucket out"=w285:T1, "Span"=w288:dbl, "time interval"=w287:T12)  [unwired: 6 in]
        n156 = Bundle By Name(cluster=w295, "Time Interval"=w287) -> (w298:T10)
        n157 = property on="Span" class="DigNum (strict)"("Value"=w288) -> ()  [unwired: 2 in, 2 out]
        n158 = local write "Time Bucket"(w285) -> ()
        n159 = call <vilib>:"Add State(s) to Queue__jki_lib_state_machine.vi"("State(s) in Front (\"\")"="Data: Write Time Interval" ("State(s) in Front (\"\")"), "State(s) in (\"\")"=w300) -> ("States Out"=w299:string)  [unwired: 13 in]
      }
      frame "Data: Write Time Interval" {
        # "Do not put any code in this frame.\n(It is a separator no-op. You can make a copy of this frame to create a new Data frame)"
        n160 = Unbundle By Name(w313) -> ("self reference"=w317:refnum<class "Database Viewer.lvclass">, "Time Interval"=w315:T12)
        n161 = Bundle By Name(cluster=w317, "Time Interval"=w315) -> (w316:refnum<class "Database Viewer.lvclass">)
        n162 = Bundle By Name(cluster=w313, "self reference"=w316) -> (w314:T10)
        n163 = call <vilib>:"Add State(s) to Queue__jki_lib_state_machine.vi"("State(s) in (\"\")"=w320) -> ("States Out"=w319:string)  [unwired: 14 in]
      }
      frame "Data: Check Connect Time" {
        w331 = timestamp(0 s since 1904-01-01)  # Connect Time
        # "Connected more than 1 hour AND not 0, disconnect"
        # "Do not put any code in this frame.\n(It is a separator no-op. You can make a copy of this frame to create a new Data frame)"
        n164 = Unbundle By Name(w332) -> ("Connect Time"=w330:timestamp)
        n165 = Not Equal?(x=w330, y=w331) -> (x != y?=w326:bool)
        n166 = Get Date/Time In Seconds() -> (seconds since 1Jan1904=w329:timestamp)
        n167 = Subtract(x=w329, y=w330) -> (x-y=w328:dbl)
        n168 = Greater?(x=w328, y=3600.0) -> (0:w325:bool)
        n169 = And(x=w325, y=w326) -> (x .and. y?=w322:bool)
        n170 = Select(t="Macro: Disconnect" ("State(s) in Front (\"\")"), s=w322, f="") -> (s? t:f=w321:string)
        n171 = call <vilib>:"Add State(s) to Queue__jki_lib_state_machine.vi"("State(s) in Front (\"\")"=w321, "State(s) in (\"\")"=w335) -> ("States Out"=w334:string)  [unwired: 13 in]
      }
      frame "Data: Update Connect Time" {
        # "Do not put any code in this frame.\n(It is a separator no-op. You can make a copy of this frame to create a new Data frame)"
        n172 = case shown="Default" w336 {
          tunnel: [timestamp(0 s since 1904-01-01) ("seconds since 1Jan1904") w344] -> w337
          frame Default {
          }
          frame "Now" {
            n173 = Get Date/Time In Seconds() -> (seconds since 1Jan1904=w344:timestamp)
          }
        }
        n174 = Bundle By Name(cluster=w339, "Connect Time"=w337) -> (w338:T10)
        n175 = call <vilib>:"Add State(s) to Queue__jki_lib_state_machine.vi"("State(s) in (\"\")"=w342) -> ("States Out"=w341:string)  [unwired: 14 in]
      }
      frame "Data: Calculate Shift Hours" {
        # "Do not put any code in this frame.\n(It is a separator no-op. You can make a copy of this frame to create a new Data frame)"
        n176 = case shown="True" "Igor" {
          tunnel: [0.0 w354] -> w345
          tunnel: "DST" -> [_ w353]
          frame False {
          }
          frame True {
            n177 = case shown="True" w353 {
              tunnel: [-5.0 -4.0] -> w354
              frame False {
              }
              frame True {
              }
            }
          }
        }
        "Shift Hours" <- w345
        n178 = call <vilib>:"Add State(s) to Queue__jki_lib_state_machine.vi"("State(s) in (\"\")"=w351) -> ("States Out"=w350:string)  [unwired: 14 in]
      }
      frame "Data: Cleanup" {
        # "Cleanup any data and references, here.\n(this is called automatically, by the Macro: Exit)"
        n179 = Unbundle By Name(w357) -> ("Core.Current VI Reference"=w360:refnum<vi>)
        n180 = Close Reference(reference=w360, error in (no error)=w359) -> (error out=w358:errorcluster)
        n181 = call <vilib>:"Add State(s) to Queue__jki_lib_state_machine.vi"("State(s) in (\"\")"=w362) -> ("States Out"=w361:string)  [unwired: 14 in]
      }
      frame "---------- UI ----------" {
        # "Do not put any code in this frame.\n(It is a separator no-op. You can make a copy of this frame to create a new UI frame)"
        n182 = call <vilib>:"Add State(s) to Queue__jki_lib_state_machine.vi"("State(s) in (\"\")"=w366) -> ("States Out"=w365:string)  [unwired: 14 in]
      }
      frame "UI: Initialize" {
        w370 = FALSE ("Load Configuration")
        w382 = "." ("Delimiter")
        w368 = string[] [] ("Value")
        w374 = string[][] [] ("Postgres Tree (Left)")
        w390 = u16[] [] ("Value")
        # "initialize with:\nend = now\nstart = now - 1 hour"
        # "Initialize the User Interface, here.\n(this is called automatically, by the Macro: Init)"
        n183 = control-ref of="postgreSQL Tree (Right / X)"() -> (w388:refnum<vi>)
        n184 = Unbundle By Name(w379) -> ("Core.Current VI Reference"=w377:refnum<vi>)
        n185 = local write "Get Trace SQL"("") -> ()
        n186 = property on="Database Time Graph" class="XYGraph (strict)"("ActXScl"=0 ("Active X Scale")) -> ()  [unwired: 2 in, 2 out]
        n187 = control-ref of="postgreSQL Tree (Left / Y)"() -> (w389:refnum<vi>)
        n188 = property on="Variables (right axis)" class="Arr (strict)"("Value"=w390) -> ()  [unwired: 2 in, 2 out]
        n189 = property on="Variables (left axis)" class="Arr (strict)"("Value"=w390) -> ()  [unwired: 2 in, 2 out]
        n190 = Get Date/Time In Seconds() -> (seconds since 1Jan1904=w395:timestamp)
        n191 = property on="Property Node" class="Tree (strict)"(reference=w389, "Value"=w368) -> (reference out=w387:refnum<vi>)  [unwired: 1 in, 1 out]
        n192 = property on="Property Node" class="Tree (strict)"(reference=w388, "Value"=w368) -> (reference out=w386:refnum<vi>)  [unwired: 1 in, 1 out]
        n193 = To Double Precision Float(number=w395) -> (double precision float=w375:dbl)
        n194 = Subtract(x=w375, y=3600.0) -> (x-y=w394:dbl)
        n195 = local write "Tab Control"(T3."Time Graph" ("Tab Control")) -> ()
        n196 = call <userlib>:"MGI Populate Tree with Delimited Strings.vi"("error in (no error)"=w385, "Delimiter"=w382, "Items (Delimited)"=w374, "Tree Control"=w387) -> ("error out"=w383:errorcluster)  [unwired: 5 in, 2 out]
        n197 = call <userlib>:"MGI Populate Tree with Delimited Strings.vi"("error in (no error)"=w385, "Delimiter"=w382, "Items (Delimited)"=w374, "Tree Control"=w386) -> ("error out"=w384:errorcluster)  [unwired: 5 in, 2 out]
        n198 = local write "End"(w375) -> ()
        n199 = local write "Start"(w394) -> ()
        n200 = Merge Errors(w383, w384) -> (w373:errorcluster)
        n201 = call <userlib>:"Fit VI window to Largest Dec__ogtk.vi"("error in (no error)"=w373, "border spacing (2 px)"=0, "VI Ref (calling VI)"=w377) -> ("error out"=w376:errorcluster, "dup VI Ref"=w372:refnum<vi>)  [unwired: 3 in]
        n202 = local write "Execute Custom SQL?"(w370) -> ()
        n203 = local write "Load Configuration"(w370) -> ()
        n204 = local write "Save Configuration"(w370) -> ()
        n205 = local write "Export Button"(w370) -> ()
        n206 = local write "Connect"(w370) -> ()
        n207 = local write "Seek Back Button"(w370) -> ()
        n208 = local write "Exit"(w370) -> ()
        n209 = local write "Seek Forward Button"(w370) -> ()
        n210 = property class="VI"(reference=w372, error in=w376, "Front Panel.PanelBounds"=T7 {"Left"=57, "Top"=141, "Right"=1385, "Bottom"=861} ("Front Panel Window:Panel Bounds")) -> (error out=w369:errorcluster)  [unwired: 1 out]
        n211 = local write "Favorite"(enum16{"A", "B", "C"}."A" ("Favorite")) -> ()
        n212 = local write "Mode"(Time_Mode--enum."Start, Now (live)" ("Mode")) -> ()
        n213 = call <vilib>:"Add State(s) to Queue__jki_lib_state_machine.vi"("State(s) in (\"\")"=w397) -> ("States Out"=w396:string)  [unwired: 14 in]
      }
      frame "UI: Cursor Set" {
        # "Argument"
        # "Set and Unset Cursor Busy.\n(Usage: \"UI: Cursor Set >> Busy|Idle\")"
        n214 = case shown="\"Busy\"" w398 {
          tunnel: w400 -> [w405 w407]
          tunnel: [w404 w406] -> w399
          frame "Idle", Default {
            n215 = call <vilib>:"Unset Busy.vi"("error in (no error)"=w405) -> ("error out"=w404:errorcluster)  [unwired: 10 in]
          }
          frame "Busy" {
            n216 = call <vilib>:"Set Busy.vi"("error in (no error)"=w407) -> ("error out"=w406:errorcluster)  [unwired: 9 in, 1 out]
          }
        }
        n217 = call <vilib>:"Add State(s) to Queue__jki_lib_state_machine.vi"("State(s) in (\"\")"=w403) -> ("States Out"=w402:string)  [unwired: 14 in]
      }
      frame "UI: Front Panel State" {
        # "Argument"
        # "Set Front Panel Open or Closed\n(Usage: \"UI: Front Panel State >> Open|Close\")"
        n218 = Unbundle By Name(w410) -> ("Core.Current VI Reference"=w409:refnum<vi>)
        n219 = case shown="\"Hidden\", \"Hide\"" w408 {
          tunnel: w412 -> [w420 w435 w446 w459 w472]
          tunnel: [w422 w436 w448 w461 w474] -> w411
          tunnel: w409 -> [w421 w433 w447 w460 w473]
          frame "Open", "Standard", Default {
            w415 = T5."Standard" ("State")
            n220 = property class="VI"(reference=w421, error in=w420) -> (reference out=w418:refnum<vi>, error out=w419:errorcluster, "FP.State"=w417:T5)
            n221 = Not Equal?(x=w417, y=w415) -> (x != y?=w416:bool)
            n222 = case shown="True" w416 {
              tunnel: [w426 w428] -> w422
              tunnel: w419 -> [w425 w428]
              tunnel: w418 -> [w424 _]
              tunnel: w415 -> [w423 _]
              frame True {
                n223 = invoke class="VI" method="FP.Open"(reference=w424, error in=w425, "Activate"=TRUE, "State"=w423) -> (error out=w426:errorcluster)  [unwired: 1 in, 4 out]
              }
              frame False {
              }
            }
          }
          frame "Close", "Closed" {
            n224 = property class="VI"(reference=w433, error in=w435) -> (reference out=w432:refnum<vi>, error out=w434:errorcluster, "FP.State"=w430:T5)
            n225 = Not Equal?(x=w430, y=T5."Closed" ("Front Panel Window:State")) -> (x != y?=w429:bool)
            n226 = case shown="True" w429 {
              tunnel: [w437 w440] -> w436
              tunnel: w434 -> [w437 w439]
              tunnel: w432 -> [_ w438]
              frame False {
              }
              frame True {
                n227 = invoke class="VI" method="FP.Close"(reference=w438, error in=w439) -> (error out=w440:errorcluster)  [unwired: 1 in, 2 out]
              }
            }
          }
          frame "Hidden", "Hide" {
            w441 = T5."Hidden" ("State")
            n228 = property class="VI"(reference=w447, error in=w446) -> (reference out=w444:refnum<vi>, error out=w445:errorcluster, "FP.State"=w443:T5)
            n229 = Not Equal?(x=w443, y=w441) -> (x != y?=w442:bool)
            n230 = case shown="True" w442 {
              tunnel: [w452 w453] -> w448
              tunnel: w445 -> [w451 w453]
              tunnel: w444 -> [w450 _]
              tunnel: w441 -> [w449 _]
              frame True {
                n231 = invoke class="VI" method="FP.Open"(reference=w450, error in=w451, "State"=w449) -> (error out=w452:errorcluster)  [unwired: 2 in, 4 out]
              }
              frame False {
              }
            }
          }
          frame "Minimize", "Minimized" {
            w454 = T5."Minimized" ("State")
            n232 = property class="VI"(reference=w460, error in=w459) -> (reference out=w457:refnum<vi>, error out=w458:errorcluster, "FP.State"=w456:T5)
            n233 = Not Equal?(x=w456, y=w454) -> (x != y?=w455:bool)
            n234 = case shown="True" w455 {
              tunnel: [w465 w466] -> w461
              tunnel: w458 -> [w464 w466]
              tunnel: w457 -> [w463 _]
              tunnel: w454 -> [w462 _]
              frame True {
                n235 = invoke class="VI" method="FP.Open"(reference=w463, error in=w464, "State"=w462) -> (error out=w465:errorcluster)  [unwired: 2 in, 4 out]
              }
              frame False {
              }
            }
          }
          frame "Maximize", "Maximized" {
            w467 = T5."Maximized" ("State")
            n236 = property class="VI"(reference=w473, error in=w472) -> (reference out=w470:refnum<vi>, error out=w471:errorcluster, "FP.State"=w469:T5)
            n237 = Not Equal?(x=w469, y=w467) -> (x != y?=w468:bool)
            n238 = case shown="True" w468 {
              tunnel: [w478 w479] -> w474
              tunnel: w471 -> [w477 w479]
              tunnel: w470 -> [w476 _]
              tunnel: w467 -> [w475 _]
              frame True {
                n239 = invoke class="VI" method="FP.Open"(reference=w476, error in=w477, "State"=w475) -> (error out=w478:errorcluster)  [unwired: 2 in, 4 out]
              }
              frame False {
              }
            }
          }
        }
        n240 = call <vilib>:"Add State(s) to Queue__jki_lib_state_machine.vi"("State(s) in (\"\")"=w414) -> ("States Out"=w413:string)  [unwired: 14 in]
      }
      frame "UI: Update Rings" {
        # "Do not put any code in this frame.\n(It is a separator no-op. You can make a copy of this frame to create a new UI frame)"
        n241 = Unbundle By Name(w481) -> ("Ring items"=w480:cluster{string, i32}[])
        n242 = property on="Ring" class="Ring (strict)"("StringsAndValues[]"=w480) -> ()  [unwired: 2 in, 2 out]
        n243 = property on="Ring" class="Ring (strict)"("StringsAndValues[]"=w480) -> ()  [unwired: 2 in, 2 out]
        n244 = call <vilib>:"Add State(s) to Queue__jki_lib_state_machine.vi"("State(s) in (\"\")"=w484) -> ("States Out"=w483:string)  [unwired: 14 in]
      }
      frame "UI: Update Graphs" {
        # "Do not put any code in this frame.\n(It is a separator no-op. You can make a copy of this frame to create a new UI frame)"
        n245 = property on="Variables (left axis)" class="Arr (strict)"() -> ("Value"=w491:u16[])  [unwired: 2 in, 2 out]
        n246 = property on="Variables (right axis)" class="Arr (strict)" props=["Value"]() -> ()  [unwired: 2 in, 3 out]
        n247 = Unbundle By Name(w492) -> ("Traces"=w488:T4)
        "Database Time Graph" <- w488
        n248 = Array Size(array=w491) -> (size(s)=w485:i32)
        n249 = Split 1D Array(array=w488, index=w485) -> (first subarray=w486:T4, second subarray=w487:T4)
        n250 = for {
          tunnel: [w499] -> w490 mode=indexing
          tunnel: w487 -> [w498] mode=indexing
          tunnel: w486 -> [w497] mode=indexing
          n251 = Unbundle By Name(w497) -> ("data"=w496:dbl[])
          n252 = Unbundle By Name(w498) -> ("data"=w495:dbl[])
          n253 = Bundle("data"=w495, "data"=w496) -> (w499:cluster{"data":dbl[], "data":dbl[]})  [unwired: 1 in]
        }
        "XY Graph" <- w490
        n254 = call <vilib>:"Add State(s) to Queue__jki_lib_state_machine.vi"("State(s) in (\"\")"=w494) -> ("States Out"=w493:string)  [unwired: 14 in]
      }
      frame "UI: Set Time Graph Y Axis" {
        # "right"
        # "left"
        # "index: # of left variable(?)"
        # "Do not put any code in this frame.\n(It is a separator no-op. You can make a copy of this frame to create a new UI frame)"
        n255 = property on="Variables (right axis)" class="Arr (strict)"() -> ("Value"=w501:u16[])  [unwired: 2 in, 2 out]
        n256 = property on="Variables (left axis)" class="Arr (strict)"() -> ("Value"=w517:u16[])  [unwired: 2 in, 2 out]
        n257 = Unbundle By Name(w523) -> ("Time Graph"=w518:refnum<vi>, "Variable Names"=w522:string[])
        n258 = Index Array(array=w517) -> (element=w521:u16)  [unwired: 1 in]
        n259 = Index Array(array=w501) -> (element=w520:u16)  [unwired: 1 in]
        n260 = Empty Array?(array=w501) -> (empty?=w519:bool)
        n261 = Array Size(array=w501) -> (size(s)=w515:i32)
        n262 = Not(x=w519) -> (.not. x?=w505:bool)
        n263 = Index Array(array=w522, index #1=w521, index #2=w520) -> (element #1=w500:string, element #2=w512:string)
        n264 = Array Size(array=w517) -> (size(s)=w506:i32)
        n265 = To Unsigned Byte Integer(number="Y Scale Mapping (Left)") -> (unsigned 8bit integer=w508:u8)
        n266 = To Unsigned Byte Integer(number="Y Scale Mapping (Right)") -> (unsigned 8bit integer=w509:u8)
        n267 = Add(x=w506, y=w515) -> (x+y=w514:i32)
        n268 = Select(t=u32 12124090, s=w505, f=u32 16448250) -> (s? t:f=w502:u32)
        n269 = property class="XYGraph (strict)"(reference=w518, "ActYScl"=0 ("Active Y Scale"), "YScale.NameLbl.Text"=w500, "YScale.Mapping Mode"=w508, "ActYScl"=1 ("Active Y Scale"), "YScale.NameLbl.Text"=w512, "YScale.Mapping Mode"=w509, "YScale.Visible"=w505, "YScale.MajGrdColor"=w502) -> (reference out=w513:refnum<vi>)  [unwired: 1 in, 1 out]
        n270 = for {
          N: w514 -> [_]
          tunnel: w506 -> [w530]
          shift-right: [w528] -> _
          shift-left: w513 -> [w527]
          i -> [w529]
          n271 = Less?(x=w530, y=w529) -> (x < y?=w531:bool)
          n272 = case shown="False" w531 {
            tunnel: w529 -> [w535 w539]
            tunnel: [w533 w536] -> w528
            tunnel: w527 -> [w532 w537]
            frame False {
              n273 = property class="XYGraph (strict)"(reference=w532, "Active Plot"=w535, "Plot.YScaleIdx"=u32 1 ("Plot.Y Scale Index")) -> (reference out=w533:refnum<vi>)  [unwired: 1 in, 1 out]
            }
            frame True {
              n274 = property class="XYGraph (strict)"(reference=w537, "Active Plot"=w539, "Plot.YScaleIdx"=u32 0 ("Plot.Y Scale Index")) -> (reference out=w536:refnum<vi>)  [unwired: 1 in, 1 out]
            }
          }
        }
        n275 = call <vilib>:"Add State(s) to Queue__jki_lib_state_machine.vi"("State(s) in (\"\")"=w526) -> ("States Out"=w525:string)  [unwired: 14 in]
      }
      frame "UI: Set Time Graph Legend" {
        # "0 & 1 indices come from here"
        # "Plot.YscaleIdx:\n0 = left\n1 = right"
        # "Do not put any code in this frame.\n(It is a separator no-op. You can make a copy of this frame to create a new UI frame)"
        n276 = property on="Variables (right axis)" class="Arr (strict)"() -> ("Value"=w548:u16[])  [unwired: 2 in, 2 out]
        n277 = property on="Variables (left axis)" class="Arr (strict)"() -> ("Value"=w549:u16[])  [unwired: 2 in, 2 out]
        n278 = Unbundle By Name(w551) -> ("Time Graph"=w550:refnum<vi>, "Variable Paths"=w543:string[])
        n279 = call "Var_Axis.vi"("Right Axis"=w548, "Left Axis"=w549) -> ("Concatenate: Left = 0, Right = 1"=w545:i32[], "Concatenate"=w547:i32[])  [unwired: 8 in]
        n280 = Array Size(array=w547) -> (size(s)=w552:i32)
        n281 = call-poly <userlib>:"Index Array Elements__ogtk.vi"("indices"=w547, "array"=w543) -> ("elements"=w544:string[])  [unwired: 9 in]
        n282 = property on="Property Node" class="XYGraph (strict)"(reference=w550, error in=w540, "LegNumRows"=w552) -> (reference out=w546:refnum<vi>, error out=w542:errorcluster)
        n283 = for {
          tunnel: w546 -> [w562]
          tunnel: w545 -> [w560] mode=indexing
          tunnel: w544 -> [w556] mode=indexing
          tunnel: w542 -> [w558]
          tunnel: [w557] -> w541
          i -> [w561]
          # "Make legend \"column: value (units)\""
          n284 = call "PG Path to Plot Label.vi"("error in (no error)"=w558, "PG Path"=w556) -> ("error out"=w559:errorcluster, "Plot Label"=w555:string)  [unwired: 7 in, 1 out]
          n285 = property on="Property Node" class="XYGraph (strict)"(reference=w562, error in=w559, "Active Plot"=w561, "Plot.YScaleIdx"=w560, "Plot.Plot Name"=w555) -> (error out=w557:errorcluster)  [unwired: 1 out]
        }
        n286 = call <vilib>:"Add State(s) to Queue__jki_lib_state_machine.vi"("State(s) in (\"\")"=w554) -> ("States Out"=w553:string)  [unwired: 14 in]
      }
      frame "UI: Set Time Graph Legend from Cursor" {
        # "Make legend \"column: value (units)\""
        # "0 & 1 indices come from here"
        # "Plot.YscaleIdx:\n0 = left\n1 = right"
        # "Do not put any code in this frame.\n(It is a separator no-op. You can make a copy of this frame to create a new UI frame)"
        n287 = property on="Variables (right axis)" class="Arr (strict)"() -> ("Value"=w573:u16[])  [unwired: 2 in, 2 out]
        n288 = property on="Variables (left axis)" class="Arr (strict)"() -> ("Value"=w574:u16[])  [unwired: 2 in, 2 out]
        n289 = Unbundle By Name(w576) -> ("Time Graph"=w575:refnum<vi>, "Variable Paths"=w568:string[], "Traces"=w564:T4)
        n290 = call "Var_Axis.vi"("Right Axis"=w573, "Left Axis"=w574) -> ("Concatenate: Left = 0, Right = 1"=w570:i32[], "Concatenate"=w572:i32[])  [unwired: 8 in]
        n291 = property on="Database Time Graph" class="XYGraph (strict)"() -> ("Cursor.Cursor X"=w563:dbl)  [unwired: 2 in, 2 out]
        n292 = Array Size(array=w572) -> (size(s)=w577:i32)
        n293 = call-poly <userlib>:"Index Array Elements__ogtk.vi"("indices"=w572, "array"=w568) -> ("elements"=w569:string[])  [unwired: 9 in]
        n294 = property on="Property Node" class="XYGraph (strict)"(reference=w575, error in=w565, "LegNumRows"=w577) -> (reference out=w571:refnum<vi>, error out=w567:errorcluster)
        n295 = for {
          tunnel: w571 -> [w596]
          tunnel: w570 -> [w594] mode=indexing
          tunnel: w569 -> [w590] mode=indexing
          tunnel: w567 -> [w592]
          tunnel: [w591] -> w566
          tunnel: w564 -> [w588] mode=indexing
          tunnel: w563 -> [w585]
          i -> [w595]
          n296 = Unbundle(w588) -> ("timestamps"=w587:timestamp[], "data"=w584:dbl[])
          n297 = To Double Precision Float(number=w587) -> (double precision float=w586:dbl[])
          n298 = Threshold 1D Array(2:w585, 3:w586) -> (0:w583:dbl)  [unwired: 1 in]
          n299 = Interpolate 1D Array(1:w583, 2:w584) -> (0:w582:dbl)
          n300 = Format Into String(format string="%.2p", w582) -> (resulting string=w581:string)  [unwired: 2 in, 1 out]
          n301 = disable-structure shown="Enabled" {
            disable-tunnel: [w600 w602] -> w593
            disable-tunnel: w592 -> [w599 w605]
            disable-tunnel: w590 -> [w598 w604]
            disable-tunnel: [w597 w603] -> w589
            disable-tunnel: w581 -> [_ w601]
            frame Disabled {
              n302 = call "PG Path to Plot Label From Cursor.vi"("error in (no error)"=w599, "PG Path"=w598) -> ("error out"=w600:errorcluster, "Plot Label"=w597:string)  [unwired: 7 in, 1 out]
            }
            frame Enabled {
              n303 = call "PG Path to Plot Label.vi"("error in (no error)"=w605, "Value"=w601, "PG Path"=w604) -> ("error out"=w602:errorcluster, "Plot Label"=w603:string)  [unwired: 6 in, 1 out]
            }
          }
          n304 = property on="Property Node" class="XYGraph (strict)"(reference=w596, error in=w593, "Active Plot"=w595, "Plot.YScaleIdx"=w594, "Plot.Plot Name"=w589) -> (error out=w591:errorcluster)  [unwired: 1 out]
        }
        n305 = call <vilib>:"Add State(s) to Queue__jki_lib_state_machine.vi"("State(s) in (\"\")"=w579) -> ("States Out"=w578:string)  [unwired: 14 in]
      }
      frame "UI: Set XY Graph Legend" {
        # "Do not put any code in this frame.\n(It is a separator no-op. You can make a copy of this frame to create a new UI frame)"
        n306 = property on="Variables (right axis)" class="Arr (strict)" props=["Value"]() -> ()  [unwired: 2 in, 3 out]
        n307 = property on="Variables (left axis)" class="Arr (strict)"() -> ("Value"=w607:u16[])  [unwired: 2 in, 2 out]
        n308 = Unbundle By Name(w615) -> ("XY Graph"=w614:refnum<vi>, "Variable Paths"=w611:string[])
        n309 = Array Size(array=w607) -> (size(s)=w606:i32)
        n310 = call-poly <userlib>:"Index Array Elements__ogtk.vi"("indices"=w607, "array"=w611) -> ("elements"=w612:string[])  [unwired: 9 in]
        n311 = property on="Property Node" class="XYGraph (strict)"(reference=w614, error in=w608, "LegNumRows"=w606) -> (reference out=w613:refnum<vi>, error out=w610:errorcluster)
        n312 = for {
          tunnel: w613 -> [w624]
          tunnel: w612 -> [w618] mode=indexing
          tunnel: w610 -> [w621]
          tunnel: [w620] -> w609
          i -> [w623]
          # "Make legend \"column: value (units)\""
          n313 = call "PG Path to Plot Label.vi"("error in (no error)"=w621, "PG Path"=w618) -> ("error out"=w622:errorcluster, "Plot Label"=w619:string)  [unwired: 7 in, 1 out]
          n314 = property on="Property Node" class="XYGraph (strict)"(reference=w624, error in=w622, "Active Plot"=w623, "Plot.Plot Name"=w619) -> (error out=w620:errorcluster)  [unwired: 1 out]
        }
        n315 = call <vilib>:"Add State(s) to Queue__jki_lib_state_machine.vi"("State(s) in (\"\")"=w617) -> ("States Out"=w616:string)  [unwired: 14 in]
      }
      frame "UI: Read Legend" {
        # "0 & 1 indices come from here"
        # "Plot.YscaleIdx:\n0 = left\n1 = right"
        # "Do not put any code in this frame.\n(It is a separator no-op. You can make a copy of this frame to create a new UI frame)"
        n316 = property on="Variables (right axis)" class="Arr (strict)"() -> ("Value"=w625:u16[])  [unwired: 2 in, 2 out]
        n317 = property on="Variables (left axis)" class="Arr (strict)"() -> ("Value"=w626:u16[])  [unwired: 2 in, 2 out]
        n318 = Unbundle By Name(w628) -> ("Time Graph"=w627:refnum<vi>)
        n319 = call "Var_Axis.vi"("Right Axis"=w625, "Left Axis"=w626) -> ()  [unwired: 8 in, 2 out]
        n320 = property on="Property Node" class="XYGraph (strict)" props=["Plot", "Point Style"](reference=w627) -> ()  [unwired: 1 in, 3 out]
        n321 = call <vilib>:"Add State(s) to Queue__jki_lib_state_machine.vi"("State(s) in (\"\")"=w631) -> ("States Out"=w630:string)  [unwired: 14 in]
      }
      frame "UI: Set XY Graph Axis Labels" {
        # "Do not put any code in this frame.\n(It is a separator no-op. You can make a copy of this frame to create a new UI frame)"
        n322 = Unbundle By Name(w643) -> ("XY Graph"=w644:refnum<vi>, "Variable Names"=w638:string[])
        n323 = property on="Variables (left axis)" class="Arr (strict)"() -> ("Value"=w639:u16[])  [unwired: 2 in, 2 out]
        n324 = property on="Variables (right axis)" class="Arr (strict)"() -> ("Value"=w640:u16[])  [unwired: 2 in, 2 out]
        n325 = for {
          tunnel: w638 -> [w651]
          tunnel: [w650] -> w637 mode=indexing
          tunnel: [w649] -> w633 mode=indexing
          tunnel: w640 -> [w648] mode=indexing
          tunnel: w639 -> [w647] mode=indexing
          n326 = Index Array(array=w651, index #1=w647, index #2=w648) -> (element #1=w650:string, element #2=w649:string)
        }
        n327 = call <userlib>:"1D Array to String__ogtk.vi"("delimiter (Tab)"=", ", "Array of Strings"=w637) -> ("delimited string"=w635:string)  [unwired: 9 in]
        n328 = call <userlib>:"1D Array to String__ogtk.vi"("delimiter (Tab)"=", ", "Array of Strings"=w633) -> ("delimited string"=w632:string)  [unwired: 9 in]
        n329 = property on="Property Node" class="XYGraph (strict)"(reference=w644, error in=w641, "YScale.NameLbl.Text"=w635, "XScale.NameLbl.Text"=w632) -> (error out=w642:errorcluster)  [unwired: 1 out]
        n330 = call <vilib>:"Add State(s) to Queue__jki_lib_state_machine.vi"("State(s) in (\"\")"=w646) -> ("States Out"=w645:string)  [unwired: 14 in]
      }
      frame "UI: Hide/show trees" {
        (unwired) T7 {"Left"=57, "Top"=141, "Right"=1385, "Bottom"=861} ("Front Panel Window:Panel Bounds")
        # "Do not put any code in this frame.\n(It is a separator no-op. You can make a copy of this frame to create a new UI frame)"
        n331 = Unbundle By Name(w667) -> ("Core.Current VI Reference"=w655:refnum<vi>)
        n332 = property on="Trees Visible? >>>>>>" class="Bool (strict)"() -> ("Value"=w666:bool)  [unwired: 2 in, 2 out]
        n333 = property class="VI"(reference=w655, error in=w669) -> (reference out=w659:refnum<vi>, error out=w660:errorcluster, "Front Panel.PanelBounds"=w656:T7)
        n334 = Unbundle By Name(w656) -> ("Right"=w658:i16)
        n335 = Less?(x=w658, y=i16 1500) -> (x < y?=w657:bool)
        n336 = Select(t=i16 0 ("Right"), s=w657, f=i16 -512 ("Right")) -> (s? t:f=w654:i16)
        n337 = Select(t=i16 512 ("Right"), s=w666, f=w654) -> (s? t:f=w664:i16)
        n338 = Add(x=w658, y=w664) -> (x+y=w652:i16)
        n339 = Bundle By Name(cluster=w656, "Right"=w652) -> (w661:T7)
        n340 = property class="VI"(reference=w659, error in=w660, "Front Panel.PanelBounds"=w661) -> (error out=w668:errorcluster)  [unwired: 1 out]
        n341 = call <vilib>:"Add State(s) to Queue__jki_lib_state_machine.vi"("State(s) in (\"\")"=w671) -> ("States Out"=w670:string)  [unwired: 14 in]
      }
      frame "UI: Show Connect Buttons" {
        # "Do not put any code in this frame.\n(It is a separator no-op. You can make a copy of this frame to create a new UI frame)"
        n342 = case shown="\"Connect\", Default" w674 {
          tunnel: [FALSE TRUE] -> w673
          tunnel: [TRUE FALSE] -> w672
          frame "Disconnect" {
          }
          frame "Connect", Default {
          }
        }
        n343 = property on="Connect" class="Bool (strict)"("Visible"=w673) -> ()  [unwired: 2 in, 2 out]
        n344 = property on="Disconnect" class="Bool (strict)"("Visible"=w672) -> ()  [unwired: 2 in, 2 out]
        n345 = call <vilib>:"Add State(s) to Queue__jki_lib_state_machine.vi"("State(s) in (\"\")"=w678) -> ("States Out"=w677:string)  [unwired: 14 in]
      }
      frame "UI: Update Status" {
        # "Do not put any code in this frame.\n(It is a separator no-op. You can make a copy of this frame to create a new UI frame)"
        n346 = case shown="\"Connected\"" w683 {
          tunnel: [u32 56327 u32 16711680] -> w686
          frame "Connected" {
          }
          frame Default {
          }
        }
        n347 = property on="Status" class="Str"("Text.TextColor"=w686) -> ()  [unwired: 2 in, 2 out]
        n348 = Bundle By Name(cluster=w685, "Status"=w683) -> (w684:T10)
        n349 = disable-structure shown="Disabled" {
          frame Disabled {
            n350 = call "Display Message to User2"() -> ()  [unwired: 10 in, 2 out]
          }
          frame Enabled {
          }
        }
        n351 = call <vilib>:"Add State(s) to Queue__jki_lib_state_machine.vi"("State(s) in (\"\")"=w689) -> ("States Out"=w688:string)  [unwired: 14 in]
        "Status" <- w683
      }
      frame "---------- Macro ----------" {
        # "Do not put any code in this frame.\n(It is a separator no-op. You can make a copy of this frame to create a new Macro frame)"
        n352 = call <vilib>:"Add State(s) to Queue__jki_lib_state_machine.vi"("State(s) in (\"\")"=w695) -> ("States Out"=w694:string)  [unwired: 14 in]
      }
      frame "Macro: Initialize" {
        # "Initialization Macro\n(This is called once, when the VI starts)"
        n353 = call <vilib>:"Add State(s) to Queue__jki_lib_state_machine.vi"("State(s) in Front (\"\")"="Data: Initialize\nInitialize Core Data\nUI: Initialize\nUI: Show Connect Buttons >> Connect\nUI: Update Status >> Disconnected\nUI: Front Panel State >> Open\nUI: Hide/show trees\nMacro: Connect\nMacro: Load Config\nMacro: Update Graph", "State(s) in (\"\")"=w700) -> ("States Out"=w699:string)  [unwired: 13 in]
      }
      frame "Macro: Connect" {
        # "Do not put any code in this frame.\n(It is a separator no-op. You can make a copy of this frame to create a new Macro frame)"
        n354 = call <vilib>:"Add State(s) to Queue__jki_lib_state_machine.vi"("State(s) in Front (\"\")"="Postgres: Open Connection\nUI: Update Status >> Connected\nUI: Show Connect Buttons >> Disconnect\nData: Update Connect Time >> Now\nPostgres: Get Tables\nPostgres: Get Variables\nUI: Update Rings" ("State(s) in Front (\"\")"), "State(s) in (\"\")"=w705) -> ("States Out"=w704:string)  [unwired: 13 in]
      }
      frame "Macro: Disconnect" {
        # "Do not put any code in this frame.\n(It is a separator no-op. You can make a copy of this frame to create a new Macro frame)"
        n355 = call <vilib>:"Add State(s) to Queue__jki_lib_state_machine.vi"("State(s) in Front (\"\")"="Postgres: Close Connection\nUI: Update Status >> Disconnected\nUI: Show Connect Buttons >> Connect\nData: Update Connect Time" ("State(s) in Front (\"\")"), "State(s) in (\"\")"=w710) -> ("States Out"=w709:string)  [unwired: 13 in]
      }
      frame "Macro: Save Config" {
        # "Initialization Macro\n(This is called once, when the VI starts)"
        n356 = call <vilib>:"Build State String with Arguments__JKI_lib_State_Machine.vi"("Arguments (\"\")"=w713, "State"="Configuration: Initialize") -> ("State with Arguments"=w712:string)  [unwired: 4 in]
        n357 = call <vilib>:"Add State(s) to Queue__jki_lib_state_machine.vi"("State(s) in Front (\"\")"=w712, "State(s) at Back (\"\")"="Configuration: Get UI Controls\nConfiguration: Write") -> ("States Out"=w711:string)  [unwired: 13 in]
        n358 = call <vilib>:"Add State(s) to Queue__jki_lib_state_machine.vi"("State(s) in Front (\"\")"=w711, "State(s) in (\"\")"=w719) -> ("States Out"=w718:string)  [unwired: 13 in]
      }
      frame "Macro: Load Config" {
        # "Initialization Macro\n(This is called once, when the VI starts)"
        n359 = call <vilib>:"Build State String with Arguments__JKI_lib_State_Machine.vi"("Arguments (\"\")"=w722, "State"="Configuration: Initialize") -> ("State with Arguments"=w723:string)  [unwired: 4 in]
        n360 = call <vilib>:"Add State(s) to Queue__jki_lib_state_machine.vi"("State(s) in Front (\"\")"=w723, "State(s) at Back (\"\")"="Configuration: Read\nConfiguration: Set UI Controls") -> ("States Out"=w720:string)  [unwired: 13 in]
        n361 = call <vilib>:"Add State(s) to Queue__jki_lib_state_machine.vi"("State(s) in Front (\"\")"=w720, "State(s) in (\"\")"=w728) -> ("States Out"=w727:string)  [unwired: 13 in]
      }
      frame "Macro: Update Graph" {
        # "Do not put any code in this frame.\n(It is a separator no-op. You can make a copy of this frame to create a new Macro frame)"
        n362 = Select(t="Database: Get Traces (SQL)" ("State(s) in Front (\"\")"), s="Execute Custom SQL?", f="Data: Get Time Interval (mode)\nDatabase: Get Traces" ("State(s) in Front (\"\")")) -> (s? t:f=w732:string)
        n363 = call <vilib>:"Add State(s) to Queue__jki_lib_state_machine.vi"("State(s) in (\"\")"=w732, "State(s) at Back (\"\")"="UI: Set Time Graph Legend from Cursor\nUI: Update Graphs" ("State(s) in Front (\"\")")) -> ("States Out"=w730:string)  [unwired: 13 in]
        n364 = call <vilib>:"Add State(s) to Queue__jki_lib_state_machine.vi"("State(s) in Front (\"\")"=w730, "State(s) in (\"\")"=w738) -> ("States Out"=w737:string)  [unwired: 13 in]
      }
      frame "Macro: Exit" {
        # "Exit Macro\n(This is called once, when the VI exits)"
        n365 = Unbundle By Name(w746) -> ("Core.Close Panel on Exit?"=w745:bool)
        n366 = Select(t="UI: Front Panel State >> Close", s=w745, f="") -> (s? t:f=w742:string)
        n367 = call <vilib>:"Add State(s) to Queue__jki_lib_state_machine.vi"("State(s) in Front (\"\")"="Macro: Save Config\nMacro: Disconnect", "State(s) in (\"\")"=w742, "State(s) at Back (\"\")"="Data: Cleanup\nExit") -> ("States Out"=w740:string)  [unwired: 12 in]
        n368 = call <vilib>:"Add State(s) to Queue__jki_lib_state_machine.vi"("State(s) in Front (\"\")"=w740, "State(s) in (\"\")"=w749) -> ("States Out"=w748:string)  [unwired: 13 in]
      }
      frame "---------- Postgres ----------" {
        # "Template Separator\n(You can make a copy of, or modify, this frame)"
        n369 = call <vilib>:"Add State(s) to Queue__jki_lib_state_machine.vi"("State(s) in (\"\")"=w753) -> ("States Out"=w752:string)  [unwired: 14 in]
      }
      frame "Postgres: Open Connection" {
        # "Template Separator\n(You can make a copy of, or modify, this frame)"
        n370 = Unbundle By Name(w761) -> ("self reference"=w757:refnum<class "Database Viewer.lvclass">)
        n371 = Unbundle By Name(w757) -> ("PG"=w756:refnum<class "LV-Data.PGSQL.lvclass">)
        n372 = call <userlib>:"PGSQL.Open.vi"("error in (no error)"=w755, "Connection String"="user = reader", "Data.PG in"=w756) -> ("error out"=w760:errorcluster, "Data.PG out"=w759:refnum<class "LV-Data.PGSQL.lvclass">)  [unwired: 7 in]
        n373 = Bundle By Name(cluster=w757, "PG"=w759) -> (w758:refnum<class "Database Viewer.lvclass">)
        n374 = Bundle By Name(cluster=w761, "self reference"=w758) -> (w762:T10)
        n375 = call <vilib>:"Add State(s) to Queue__jki_lib_state_machine.vi"("State(s) in (\"\")"=w764) -> ("States Out"=w763:string)  [unwired: 14 in]
      }
      frame "Postgres: Get Tables" {
        # "Template Separator\n(You can make a copy of, or modify, this frame)"
        n376 = Unbundle By Name(w770) -> ("self reference"=w768:refnum<class "Database Viewer.lvclass">)
        n377 = Unbundle By Name(w768) -> ("PG"=w766:refnum<class "LV-Data.PGSQL.lvclass">)
        n378 = call <userlib>:"List Tables.vi"("error in (no error)"=w772, "Data.PG"=w766) -> ("error out"=w771:errorcluster, "Table Paths"=w765:string[], "Table Names"=w773:string[], "Data.PG"=w769:refnum<class "LV-Data.PGSQL.lvclass">)  [unwired: 6 in]
        n379 = Bundle By Name(cluster=w768, "PG"=w769) -> (w767:refnum<class "Database Viewer.lvclass">)
        n380 = Bundle By Name(cluster=w770, "self reference"=w767, "PG Variables.Table Names"=w773, "PG Variables.Table Paths"=w765) -> (w774:T10)
        n381 = call <vilib>:"Add State(s) to Queue__jki_lib_state_machine.vi"("State(s) in (\"\")"=w776) -> ("States Out"=w775:string)  [unwired: 14 in]
      }
      frame "Postgres: Get Variables" {
        # "Template Separator\n(You can make a copy of, or modify, this frame)"
        n382 = Unbundle By Name(w780) -> ("self reference"=w778:refnum<class "Database Viewer.lvclass">, "PG Variables.Table Paths"=w788:string[], "PG Variables.Table Names"=w787:string[])
        n383 = Unbundle By Name(w778) -> ("PG"=w779:refnum<class "LV-Data.PGSQL.lvclass">)
        n384 = for {
          tunnel: w788 -> [w794] mode=indexing
          tunnel: w779 -> [w801]
          tunnel: w787 -> [w803] mode=indexing
          tunnel: [w796] -> w786 mode=concatenating
          tunnel: [w802] -> w784 mode=concatenating
          tunnel: w782 -> [w798]
          tunnel: [w795] -> w781
          shift-right: [w791] -> w777
          shift-left: w778 -> [w793]
          n385 = call <userlib>:"List Columns.vi"("error in (no error)"=w798, "Table Path"=w794, "Data.PG"=w801) -> ("error out"=w795:errorcluster, "Column Paths"=w799:string[], "Column Names"=w800:string[], "Data.PG out"=w792:refnum<class "LV-Data.PGSQL.lvclass">, "Column Units"=w797:string[])  [unwired: 4 in]
          n386 = for {
            tunnel: w799 -> [w813] mode=indexing
            tunnel: w794 -> [w812]
            tunnel: w803 -> [w807]
            tunnel: w800 -> [w806] mode=indexing
            tunnel: w797 -> [w805] mode=indexing
            tunnel: [w811] -> w796 mode=indexing
            tunnel: [w804] -> w802 mode=indexing
            n387 = call <userlib>:"Build Path.vi"("Table path"=w812, "Column path"=w813, "Table name"=w807, "Column name"=w806, "Column units"=w805) -> ("PG path"=w811:string)  [unwired: 10 in]
            n388 = Concatenate Strings(w807, ": " ("string"), w806, " (" ("string"), w805, ")" ("string")) -> (w804:string)
          }
          n389 = Bundle By Name(cluster=w793, "PG"=w792) -> (w791:refnum<class "Database Viewer.lvclass">)
        }
        n390 = Bundle By Name(cluster=w780, "self reference"=w777, "PG Variables.PG Columns"=w786, "PG Variables.PG Names"=w784) -> (w783:T10)
        n391 = call <vilib>:"Add State(s) to Queue__jki_lib_state_machine.vi"("State(s) in Front (\"\")"="Postgres: Add Variables" ("State(s) in Front (\"\")"), "State(s) in (\"\")"=w790) -> ("States Out"=w789:string)  [unwired: 13 in]
      }
      frame "Postgres: Add Variables" {
        w828 = FALSE
        w830 = ":" ("Delimiter")
        # "Template Separator\n(You can make a copy of, or modify, this frame)"
        n392 = Unbundle By Name(w825) -> ("Variable Paths"=w817:string[], "PG Variables.PG Columns"=w816:string[], "Variable Names"=w814:string[], "PG Variables.PG Names"=w815:string[])
        n393 = Insert Into Array(array=w817, new element=w816) -> (w835:string[])  [unwired: 1 in]
        n394 = Insert Into Array(array=w814, new element=w815) -> (w836:string[])  [unwired: 1 in]
        n395 = control-ref of="postgreSQL Tree (Left / Y)"() -> (w833:refnum<vi>)
        n396 = control-ref of="postgreSQL Tree (Right / X)"() -> (w832:refnum<vi>)
        n397 = for {
          tunnel: w836 -> [w840] mode=indexing
          tunnel: [w841] -> w818 mode=indexing
          tunnel: [w839] -> w831 mode=indexing
          i -> [w842]
          n398 = Bundle(w840, w842) -> (w841:cluster{string, i32})  [unwired: 1 in]
          n399 = Build Array(w840, w840) -> (w839:string[])
        }
        n400 = call <userlib>:"MGI Populate Tree with Delimited Strings.vi"("error in (no error)"=w819, "Delimiter"=w830, "Items (Delimited)"=w831, "Tree Control"=w833) -> ("error out"=w829:errorcluster, "Tree Control Dup"=w821:refnum<vi>)  [unwired: 5 in, 1 out]
        n401 = call <userlib>:"MGI Populate Tree with Delimited Strings.vi"("error in (no error)"=w819, "Delimiter"=w830, "Items (Delimited)"=w831, "Tree Control"=w832) -> ("error out"=w827:errorcluster, "Tree Control Dup"=w820:refnum<vi>)  [unwired: 5 in, 1 out]
        n402 = invoke on="Invoke Node" class="Tree" method="Open/Close.Open/Close All"(reference=w820, error in=w827, "Open"=w828) -> (error out=w822:errorcluster)  [unwired: 1 in, 3 out]
        n403 = invoke on="Invoke Node" class="Tree" method="Open/Close.Open/Close All"(reference=w821, error in=w829, "Open"=w828) -> (error out=w823:errorcluster)  [unwired: 1 in, 3 out]
        n404 = Bundle By Name(cluster=w825, "Variable Paths"=w835, "Variable Names"=w836, "Ring items"=w818) -> (w826:T10)
        n405 = call <vilib>:"Add State(s) to Queue__jki_lib_state_machine.vi"("State(s) in Front (\"\")"="UI: Update Rings" ("State(s) in Front (\"\")"), "State(s) in (\"\")"=w838) -> ("States Out"=w837:string)  [unwired: 13 in]
        n406 = Merge Errors(w823, w822) -> (w824:errorcluster)
      }
      frame "Postgres: Tree (left)" {
        # "Template Separator\n(You can make a copy of, or modify, this frame)"
        n407 = Unbundle By Name(w843) -> ("Variable Names"=w846:string[])
        n408 = property on="postgreSQL Tree (Left / Y)" class="Tree (strict)"() -> ("Value"=w845:string[])  [unwired: 2 in, 2 out]
        n409 = for {
          tunnel: w846 -> [w854]
          tunnel: w845 -> [w852] mode=indexing
          tunnel: [w853] -> w844 mode=indexing if=w850
          n410 = Search 1D Array(1D array=w854, element=w852) -> (index of element=w853:i32)  [unwired: 1 in]
          n411 = call <userlib>:"MGI String Pattern Match Exists.vi"("Patterns to Try"=string[] [":"], "String"=w852) -> ("Match Found"=w850:bool)  [unwired: 1 out]
        }
        n412 = property on="Variables (left axis)" class="Arr (strict)"("Val(Sgnl)"=w844) -> ()  [unwired: 2 in, 2 out]
        n413 = call <vilib>:"Add State(s) to Queue__jki_lib_state_machine.vi"("State(s) in (\"\")"=w849) -> ("States Out"=w848:string)  [unwired: 14 in]
      }
      frame "Postgres: Tree (right)" {
        # "Template Separator\n(You can make a copy of, or modify, this frame)"
        n414 = Unbundle By Name(w858) -> ("Variable Names"=w857:string[])
        n415 = property on="postgreSQL Tree (Right / X)" class="Tree (strict)"() -> ("Value"=w856:string[])  [unwired: 2 in, 2 out]
        n416 = for {
          tunnel: w857 -> [w866]
          tunnel: w856 -> [w864] mode=indexing
          tunnel: [w865] -> w855 mode=indexing if=w862
          n417 = Search 1D Array(1D array=w866, element=w864) -> (index of element=w865:i32)  [unwired: 1 in]
          n418 = call <userlib>:"MGI String Pattern Match Exists.vi"("Patterns to Try"=string[] [":"], "String"=w864) -> ("Match Found"=w862:bool)  [unwired: 1 out]
        }
        n419 = property on="Variables (right axis)" class="Arr (strict)"("Val(Sgnl)"=w855) -> ()  [unwired: 2 in, 2 out]
        n420 = call <vilib>:"Add State(s) to Queue__jki_lib_state_machine.vi"("State(s) in (\"\")"=w861) -> ("States Out"=w860:string)  [unwired: 14 in]
      }
      frame "Postgres: Close Connection" {
        # "Template Separator\n(You can make a copy of, or modify, this frame)"
        n421 = Unbundle By Name(w871) -> ("self reference"=w868:refnum<class "Database Viewer.lvclass">)
        n422 = Unbundle By Name(w868) -> ("PG"=w870:refnum<class "LV-Data.PGSQL.lvclass">)
        n423 = call-dynamic "Close.vi"("error in (no error)"=w874, "Data.PG in"=w870) -> ("error out"=w873:errorcluster, "Data.PG out"=w869:refnum<class "LV-Data.PGSQL.lvclass">)  [unwired: 8 in]
        n424 = Bundle By Name(cluster=w868, "PG"=w869) -> (w867:refnum<class "Database Viewer.lvclass">)
        n425 = Bundle By Name(cluster=w871, "self reference"=w867) -> (w872:T10)
        n426 = call <vilib>:"Add State(s) to Queue__jki_lib_state_machine.vi"("State(s) in (\"\")"=w876) -> ("States Out"=w875:string)  [unwired: 14 in]
      }
      frame "---------- Database ----------" {
        # "Template Separator\n(You can make a copy of, or modify, this frame)"
        n427 = call <vilib>:"Add State(s) to Queue__jki_lib_state_machine.vi"("State(s) in (\"\")"=w880) -> ("States Out"=w879:string)  [unwired: 14 in]
      }
      frame "Database: Get Traces" {
        # "Your code here.\n(You can make a copy of, or modify, this frame)"
        n428 = local read "Median Filter?"() -> (w886:bool)
        n429 = property on="Max Points" class="DigNum (strict)"() -> ("Value"=w892:i32)  [unwired: 2 in, 2 out]
        n430 = property on="Variables (left axis)" class="Arr (strict)"() -> ("Value"=w905:u16[])  [unwired: 2 in, 2 out]
        n431 = property on="Variables (right axis)" class="Arr (strict)"() -> ("Value"=w904:u16[])  [unwired: 2 in, 2 out]
        n432 = Unbundle By Name(w903) -> ("self reference"=w889:refnum<class "Database Viewer.lvclass">, "Variable Paths"=w895:string[])
        n433 = call "Var_Axis.vi"("Right Axis"=w904, "Left Axis"=w905) -> ("Concatenate"=w902:i32[])  [unwired: 8 in, 1 out]
        n434 = call-poly <userlib>:"Index Array Elements__ogtk.vi"("indices"=w902, "array"=w895) -> ("elements"=w893:string[])  [unwired: 9 in]
        n435 = for {
          tunnel: w893 -> [w914] mode=indexing
          tunnel: "Time Bucket" -> [w925]
          tunnel: [w921] -> w890 mode=indexing
          tunnel: [w918] -> w900 mode=indexing
          tunnel: w894 -> [w926]
          tunnel: [w922] -> w898
          tunnel: w892 -> [w927]
          tunnel: [w920] -> _ mode=indexing
          shift-right: [w915] -> w888
          shift-left: w889 -> [w919]
          tunnel: [w913] -> w885 mode=indexing
          tunnel: [w912] -> w884 mode=indexing
          tunnel: [w909] -> w881
          n436 = call "Construct SQL.vi"("Time Bucket"=w925, "max points"=w927, "error in (no error)"=w926, "PG path"=w914, "Database Viewer"=w919) -> ("error out"=w924:errorcluster, "SQL string"=w918:string, "Database Viewer out"=w917:refnum<class "Database Viewer.lvclass">, "Time Bucket out"=w909:T1)  [unwired: 3 in]
          n437 = call "Execute SQL.vi"("error in (no error)"=w924, "SQL string"=w918, "Database Viewer"=w917) -> ("error out"=w923:errorcluster, "SQL Result"=w910:string[][], "Database Viewer out"=w916:refnum<class "Database Viewer.lvclass">)  [unwired: 6 in]
          n438 = call "SQL Results to Trace.vi"("error in (no error)"=w923, "Result"=w910, "PG Path"=w914, "Database Viewer"=w916) -> ("error out"=w922:errorcluster, "Latest Value"=w920:string, "Trace"=w921:cluster{timestamp[], dbl[]}, "Database Viewer out"=w915:refnum<class "Database Viewer.lvclass">)  [unwired: 4 in]
          n439 = Index Array(array=w910, index (col) #1=0 ("disabled index (col)")) -> (element #1=w913:string[], element #2=w912:string[])  [unwired: 3 in]
        }
        n440 = local write "Time Bucket"(w881) -> ()
        n441 = Build Array (concatenate)(w885, w884) -> (w883:string[][])
        n442 = call "Filter Traces.vi"("error in (no error)"=w898, "Median Filter?"=w886, "Array"=w890, "Database Viewer in"=w888) -> ("error out"=w897:errorcluster, "Database Trace out"=w896:T4, "Database Viewer out"=w887:refnum<class "Database Viewer.lvclass">)  [unwired: 5 in]
        n443 = Transpose 2D Array(2D array=w883) -> (transposed array=w882:string[][])
        n444 = local write "SQL Result"(w882) -> ()
        n445 = Bundle By Name(cluster=w903, "self reference"=w887, "Traces"=w896) -> (w906:T10)
        n446 = call <userlib>:"1D Array to String__ogtk.vi"("delimiter (Tab)"="\n", "Array of Strings"=w900) -> ("delimited string"=→"Get Trace SQL":string)  [unwired: 9 in]
        n447 = call <vilib>:"Add State(s) to Queue__jki_lib_state_machine.vi"("State(s) in (\"\")"=w908) -> ("States Out"=w907:string)  [unwired: 14 in]
      }
      frame "Database: Get Traces (SQL)" {
        # "Your code here.\n(You can make a copy of, or modify, this frame)"
        n448 = Unbundle By Name(w943) -> ("self reference"=w937:refnum<class "Database Viewer.lvclass">)
        n449 = call "Execute SQL.vi"("error in (no error)"=w935, "SQL string"="SQL String", "Database Viewer"=w937) -> ("error out"=w933:errorcluster, "SQL Result"=w929:string[][], "Database Viewer out"=w934:refnum<class "Database Viewer.lvclass">)  [unwired: 6 in]
        "SQL Result" <- w929
        n450 = call "SQL Results to Trace.vi"("error in (no error)"=w933, "Result"=w929, "Database Viewer"=w934) -> ("error out"=w930:errorcluster, "Trace"=w932:cluster{timestamp[], dbl[]}, "Database Viewer out"=w928:refnum<class "Database Viewer.lvclass">)  [unwired: 5 in, 1 out]
        n451 = local read "Median Filter?"() -> (w941:bool)
        n452 = Build Array(w932) -> (w931:cluster{timestamp[], dbl[]}[])
        n453 = call "Remove Bad Points.vi"("error in (no error)"=w930, "Database Trace In"=w931) -> ("error out"=w942:errorcluster, "Database Trace Out"=w938:T4)  [unwired: 7 in, 1 out]
        n454 = case shown="True" w941 {
          tunnel: w942 -> [w947 w952]
          tunnel: [w947 w951] -> w940
          tunnel: w938 -> [w948 w950]
          tunnel: [w948 w949] -> w939
          frame False {
          }
          frame True {
            n455 = call "Median Filter.vi"("error in (no error)"=w952, "Database Trace"=w950) -> ("error out"=w951:errorcluster, "Database Trace out"=w949:T4)  [unwired: 7 in, 1 out]
          }
        }
        n456 = Bundle By Name(cluster=w943, "self reference"=w928, "Traces"=w939) -> (w944:T10)
        n457 = call <vilib>:"Add State(s) to Queue__jki_lib_state_machine.vi"("State(s) in (\"\")"=w946) -> ("States Out"=w945:string)  [unwired: 14 in]
      }
      frame "Database: Database Trace" {
        # "Template Separator\n(You can make a copy of, or modify, this frame)"
        n458 = Unbundle By Name(w955) -> ("NewRange"=w956:T9)
        n459 = Unbundle By Name(w956) -> ("Maximum"=w954:dbl, "Minimum"=w953:dbl)
        n460 = property on="End" class="DigNum (strict)"("Val(Sgnl)"=w954) -> ()  [unwired: 2 in, 2 out]
        n461 = property on="Start" class="DigNum (strict)"("Value"=w953) -> ()  [unwired: 2 in, 2 out]
        n462 = call <vilib>:"Add State(s) to Queue__jki_lib_state_machine.vi"("State(s) in (\"\")"=w959) -> ("States Out"=w958:string)  [unwired: 14 in]
      }
      frame "Database: Export" {
        w967 = T14 2 items=["User Home"=0, "User Desktop"=1, "User Documents"=2, "User Application Data"=3, "User Preferences"=4, "User Temporary"=5, "Public Documents"=6, "Public Application Data"=7, "Public Preferences"=8, "Public Cache"=13, "System Core Libraries"=9, "System Installed Libraries"=10, "Application Files"=11, "Boot Volume Root"=12] ("system directory type")
        # "Template Separator\n(You can make a copy of, or modify, this frame)"
        n463 = Unbundle By Name(w974) -> ("Time Graph"=w968:refnum<vi>)
        n464 = call <vilib>:"Get System Directory.vi"("system directory type"=w967) -> ("system directory"=w962:path)  [unwired: 10 in]
        n465 = property on="Property Node" class="XYGraph (strict)"(reference=w968, error in=w964) -> (error out=w971:errorcluster, "Value"=w973:T4)  [unwired: 1 out]
        n466 = Empty String/Path?(string/path="export path") -> (empty?=w966:bool)
        n467 = Build Path(base path=w962, name or relative path="Database Export" ("filename")) -> (appended path=w961:path)
        n468 = Select(t=w961, s=w966, f="export path") -> (s? t:f=w960:path)
        n469 = disable-structure shown="Disabled" {
          disable-tunnel: w960 -> [w979 _]
          disable-tunnel: w968 -> [w978 _]
          frame Disabled {
            # "#todo\nuse LV to ITX Export VIs"
            n470 = call <userlib>:"XY Graph to Igor Graph.vi"("XY Graph Reference"=w978, "Path"=w979) -> ()  [unwired: 8 in, 2 out]
          }
          frame Enabled {
          }
        }
        n471 = for {
          tunnel: w973 -> [w984] mode=indexing
          tunnel: [w987] -> w975 mode=indexing
          n472 = local read "Shift Hours"() -> (w981:dbl)
          n473 = Unbundle(w984) -> ("timestamps"=w988:timestamp[], "data"=w983:dbl[])
          n474 = To Double Precision Float(number=w988) -> (double precision float=w982:dbl[])
          n475 = Multiply(x=w981, y=3600.0) -> (x*y=w985:dbl)
          n476 = Add(x=w985, y=w982) -> (x+y=w986:dbl[])
          n477 = Bundle(w986, "data"=w983) -> (w987:cluster{dbl[], "data":dbl[]})  [unwired: 1 in]
        }
        n478 = local write "export path"(w960) -> ()
        n479 = Build Path(base path=w960, name or relative path="export" ("filename")) -> (appended path=w969:path)
        n480 = call <userlib>:"LV to ITX XY AutoPlot.vi"("error in"=w971, "XY-Data []"=w975, "path"=w969) -> ("error out"=w970:errorcluster)  [unwired: 7 in, 1 out]
        n481 = call <vilib>:"Add State(s) to Queue__jki_lib_state_machine.vi"("State(s) in (\"\")"=w977) -> ("States Out"=w976:string)  [unwired: 14 in]
      }
      frame "---------- Configuration ----------" {
        # "Do not put any code in this frame.\n(it is a separator no-op)"
        n482 = call <vilib>:"Add State(s) to Queue__jki_lib_state_machine.vi"("State(s) in (\"\")"=w992) -> ("States Out"=w991:string)  [unwired: 14 in]
      }
      frame "Configuration: Initialize" {
        w1001 = T14 3 items=["User Home"=0, "User Desktop"=1, "User Documents"=2, "User Application Data"=3, "User Preferences"=4, "User Temporary"=5, "Public Documents"=6, "Public Application Data"=7, "Public Preferences"=8, "Public Cache"=13, "System Core Libraries"=9, "System Installed Libraries"=10, "Application Files"=11, "Boot Volume Root"=12] ("system directory type")
        n483 = Unbundle By Name(w1006) -> ("Configuration"=w1005:refnum<class "Configuration.lvclass">)
        n484 = call <vilib>:"Get System Directory.vi"("system directory type"=w1001) -> ("system directory"=w1000:path)  [unwired: 10 in]
        n485 = Format Into String(format string="Config_%s.ini" ("File (Configuration.ini)"), error in=w996, w993) -> (resulting string=w997:string, error out=w994:errorcluster)  [unwired: 1 in]
        n486 = Build Path(base path=w1000, name or relative path="LevyLab\\Database Viewer" ("File (Configuration.ini)")) -> (appended path=w998:path)
        n487 = call <userlib>:"Write Path.vi"("error in (no error)"=w994, "Filename [Configuration.ini]"=w997, "Path"=w998, "Configuration in"=w1005) -> ("error out"=w1004:errorcluster, "Configuration out"=w1003:refnum<class "Configuration.lvclass">)  [unwired: 6 in]
        n488 = Bundle By Name(cluster=w1006, "Configuration"=w1003) -> (w1002:T10)
        n489 = call <vilib>:"Add State(s) to Queue__jki_lib_state_machine.vi"("State(s) in (\"\")"=w1008) -> ("States Out"=w1007:string)  [unwired: 14 in]
      }
      frame "Configuration: Read" {
        n490 = Unbundle By Name(w1017) -> ("Configuration"=w1018:refnum<class "Configuration.lvclass">, "Controls Cluster"=w1012:T8)
        n491 = call <userlib>:"Read Configuration.vi"("INI Fomatted Cluster Type"=w1012, "error in (no error)"=w1016, "Configuration in"=w1018) -> ("error out"=w1010:errorcluster, "Configuration"=w1013:variant, "Configuration out"=w1014:refnum<class "Configuration.lvclass">)  [unwired: 6 in]
        n492 = Variant To Data(error in=w1010, type=w1012, Variant=w1013) -> (data=w1009:T8, error out=w1011:errorcluster)
        n493 = Bundle By Name(cluster=w1017, "Configuration"=w1014, "Controls Cluster"=w1009) -> (w1015:T10)
        n494 = call <vilib>:"Add State(s) to Queue__jki_lib_state_machine.vi"("State(s) in (\"\")"=w1020) -> ("States Out"=w1019:string)  [unwired: 14 in]
      }
      frame "Configuration: Write" {
        n495 = Unbundle By Name(w1022) -> ("Configuration"=w1027:refnum<class "Configuration.lvclass">, "Controls Cluster"=w1026:T8)
        n496 = call <userlib>:"Write Configuration.vi"("error in (no error)"=w1024, "Variant"=w1026, "Configuration in"=w1027) -> ("error out"=w1023:errorcluster, "Configuration out"=w1021:refnum<class "Configuration.lvclass">)  [unwired: 7 in]
        n497 = Bundle By Name(cluster=w1022, "Configuration"=w1021) -> (w1025:T10)
        n498 = call <vilib>:"Add State(s) to Queue__jki_lib_state_machine.vi"("State(s) in (\"\")"=w1029) -> ("States Out"=w1028:string)  [unwired: 14 in]
      }
      frame "Configuration: Get UI Controls" {
        n499 = local read "Mode"() -> (w1044:T2)
        n500 = local read "Variables (left axis)"() -> (w1034:u16[])
        n501 = local read "Median Filter?"() -> (w1030:bool)
        n502 = local read "Y Scale Mapping (Left)"() -> (w1032:enum16{"linear", "log"})
        n503 = local read "Start"() -> (w1042:dbl)
        n504 = local read "Seek"() -> (w1041:dbl)
        n505 = local read "DST"() -> (w1039:bool)
        n506 = To Time Stamp(1:w1042) -> (0:w1038:timestamp)
        n507 = local read "Time Bucket"() -> (w1035:T1)
        n508 = local read "Variables (right axis)"() -> (w1033:u16[])
        n509 = local read "Max Points"() -> (w1031:i32)
        n510 = local read "Y Scale Mapping (Right)"() -> (w1043:enum16{"linear", "log"})
        n511 = local read "End"() -> (w1037:dbl)
        n512 = local read "export path"() -> (w1040:path)
        n513 = To Time Stamp(1:w1037) -> (0:w1036:timestamp)
        n514 = Bundle By Name(cluster=T8 {"Variables (left axis)"=[], "Variables (right axis)"=[], "Time Mode"=enum."Start + Span", "Time Bucket"=enum."max points", "Start Time"=timestamp(0 s since 1904-01-01), "End Time"=timestamp(0 s since 1904-01-01), "Step Size"=0.0, "Y Scale Mapping (left)"=enum."linear", "max points per trace (all)"=0, "Y Scale Mapping (right)"=enum."linear", "Filter?"=FALSE, "export path"=path "", "DST"=FALSE} ("Controls Cluster"), "Time Mode"=w1044, "Time Bucket"=w1035, "Variables (left axis)"=w1034, "Variables (right axis)"=w1033, "Filter?"=w1030, "max points per trace (all)"=w1031, "Y Scale Mapping (left)"=w1032, "Y Scale Mapping (right)"=w1043, "Start Time"=w1038, "End Time"=w1036, "Step Size"=w1041, "export path"=w1040, "DST"=w1039) -> (w1045:T8)
        n515 = Bundle By Name(cluster=w1048, "Controls Cluster"=w1045) -> (w1047:T10)
        n516 = call <vilib>:"Add State(s) to Queue__jki_lib_state_machine.vi"("State(s) in (\"\")"=w1051) -> ("States Out"=w1050:string)  [unwired: 14 in]
      }
      frame "Configuration: Set UI Controls" {
        n517 = Unbundle By Name(w1060) -> ("Controls Cluster"=w1064:T8)
        n518 = Unbundle By Name(w1064) -> ("DST"=w1063:bool, "Filter?"=w1062:bool, "export path"=w1061:path, "max points per trace (all)"=w1056:i32, "Time Mode"=w1054:T2, "Time Bucket"=w1052:T1, "Variables (left axis)"=w1055:u16[], "Variables (right axis)"=w1059:u16[], "Y Scale Mapping (left)"=w1058:enum16{"linear", "log"}, "Y Scale Mapping (right)"=w1053:enum16{"linear", "log"}, "Step Size"=w1057:dbl)
        n519 = local write "Median Filter?"(w1062) -> ()
        n520 = local write "Max Points"(w1056) -> ()
        n521 = local write "Time Bucket"(w1052) -> ()
        n522 = local write "Variables (right axis)"(w1059) -> ()
        n523 = local write "Y Scale Mapping (Right)"(w1053) -> ()
        n524 = local write "DST"(w1063) -> ()
        n525 = local write "export path"(w1061) -> ()
        n526 = local write "Mode"(w1054) -> ()
        n527 = property on="Variables (left axis)" class="Arr (strict)"("Val(Sgnl)"=w1055) -> ()  [unwired: 2 in, 2 out]
        n528 = local write "Y Scale Mapping (Left)"(w1058) -> ()
        n529 = local write "Seek"(w1057) -> ()
        n530 = call <vilib>:"Add State(s) to Queue__jki_lib_state_machine.vi"("State(s) in (\"\")"=w1067) -> ("States Out"=w1066:string)  [unwired: 14 in]
      }
    }
  }
